vi "GVSDV DOCKING.vi"(8 "sData":string, 9 "DataView Index":i32, 11 "sAction":string) -> (0 "nData_Out":i32, 1 "tWindow_Out":T3, 2 "pVIRef_Tmp":refnum<vi>, 3 "pSPRef_Out":refnum<vi>)   [LabVIEW 2013]
uses:
  <vilib>/Utility/miscctls.llb/LVBoundsTypeDef.ctl
  <vilib>/Utility/miscctls.llb/LVPositionTypeDef.ctl
  GVSNew View Global.vi
panel:
  in  "child_sp_count":i32
  in  "spliter_idx":i32
  out "Position tmp":T1
  out "Container Bounds tmp":T2
  in  "cur_panel_idx":i32
  in  "pSPRef":refnum<vi>
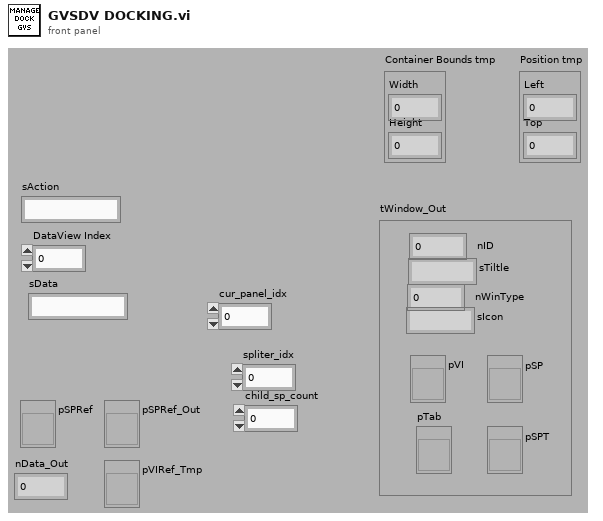
[diagram p1: front panel]
types:
  T1 = typedef "LVPositionTypeDef.ctl" = cluster{"Left":i32, "Top":i32}
  T2 = typedef "LVBoundsTypeDef.ctl" = cluster{"Width":u32, "Height":u32}
  T3 = cluster{"nID":i32, "sTiltle":string, "pVI":refnum<vi>, "pSP":refnum<vi>, "pTab":refnum<vi>, "pSPT":refnum<vi>, "nWinType":i32, "sIcon":string}
  T4 = typedef "Graph Main Info Cluster.ctl" = cluster{"Selected_BarIdx":i32, "Selected_PanelIdx":i32, "Graph Main VIRef":refnum<vi>, "ToolBarClick":bool, "Spliter Ref Array":refnum<vi>[], "Panel Ref Array":refnum<vi>[], "Spliter_matrix":i32[][], "Panel_matrix":i32[][], "child_spliterIdx_matrix":i32[][], "split_pos_matrix":i32[][], "Title State":bool, "sQueueName":string, "Frame nID":i32, "Graph VIRef Array":cluster{"Graph VIRef":refnum<vi>, "Panel Idx":i32, "Frame VIRef":refnum<vi>, "Icon Ring":i32, "Graph Type":string}[], "View Type":string}
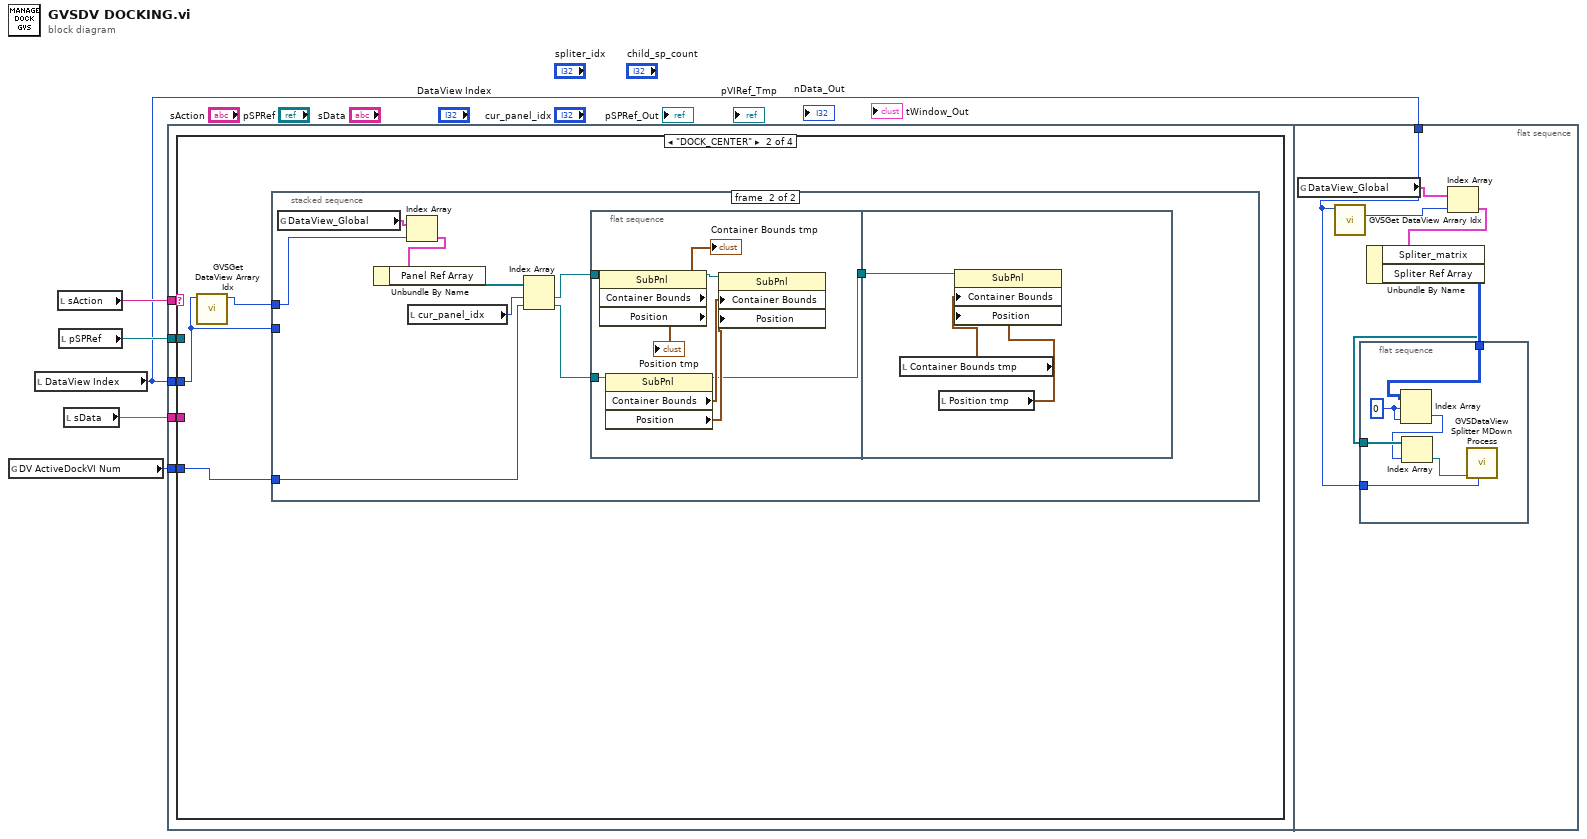
[diagram p0: block diagram]
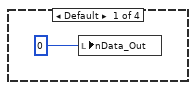
[diagram p2: hidden frame]
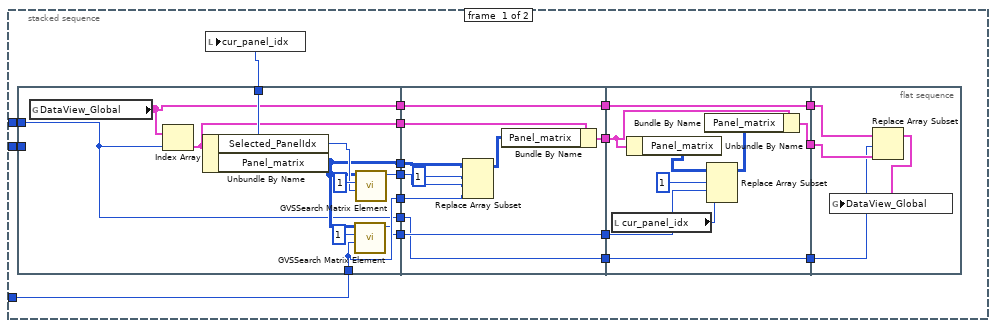
[diagram p3: hidden frame]
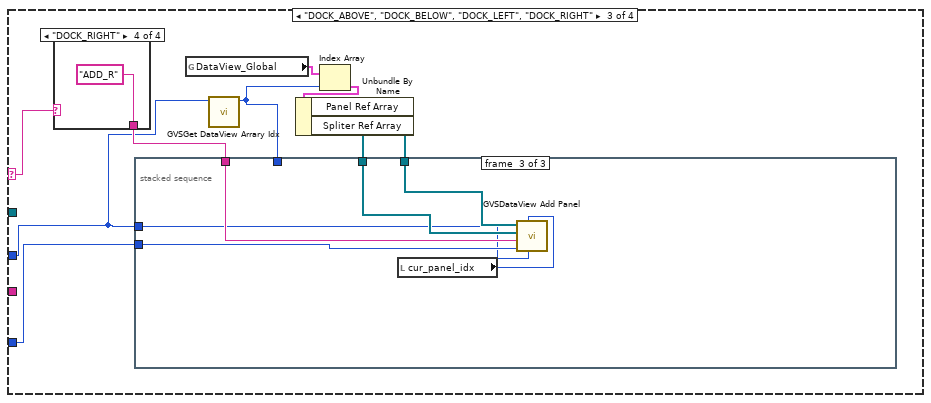
[diagram p4: hidden frame]
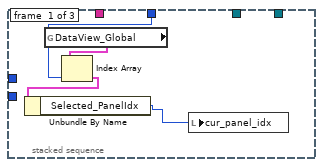
[diagram p5: hidden frame]
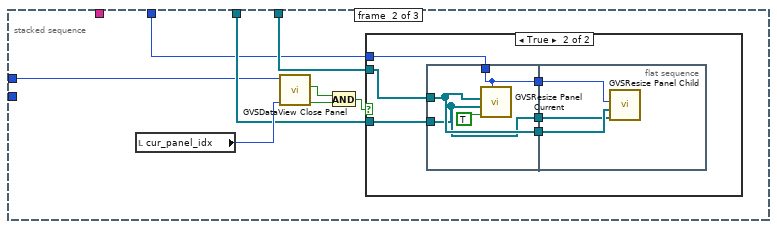
[diagram p6: hidden frame]
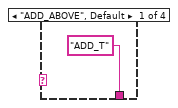
[diagram p8: hidden frame]
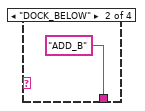
[diagram p9: hidden frame]
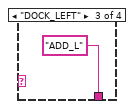
[diagram p10: hidden frame]
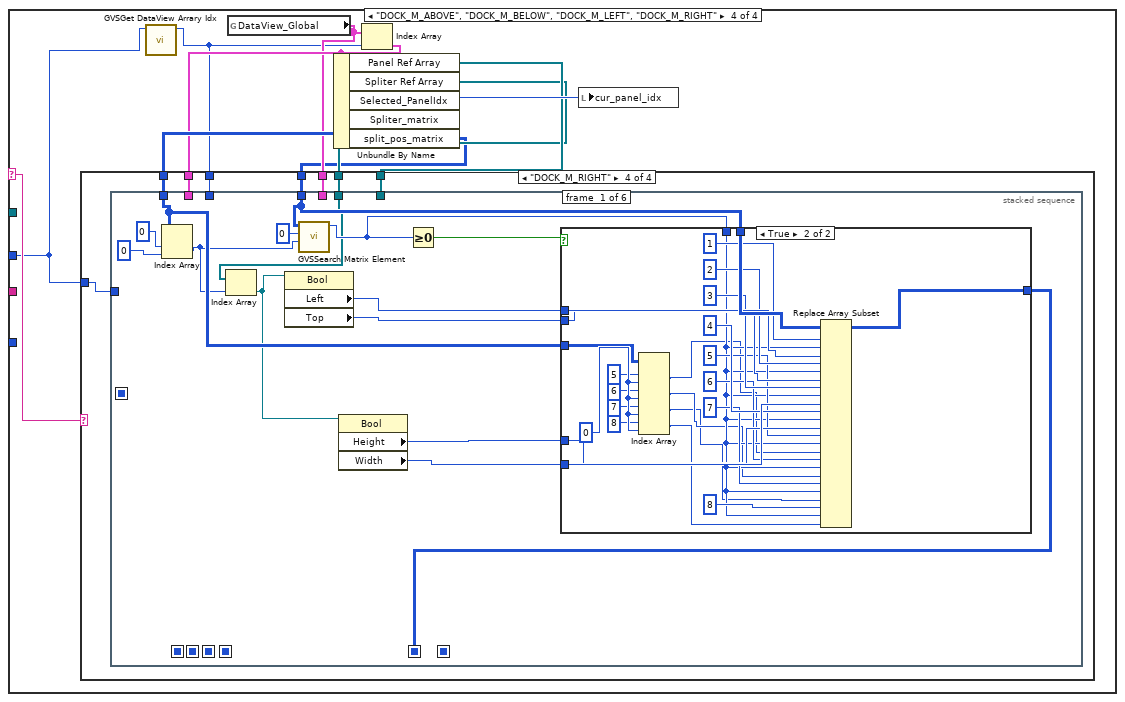
[diagram p11: hidden frame]
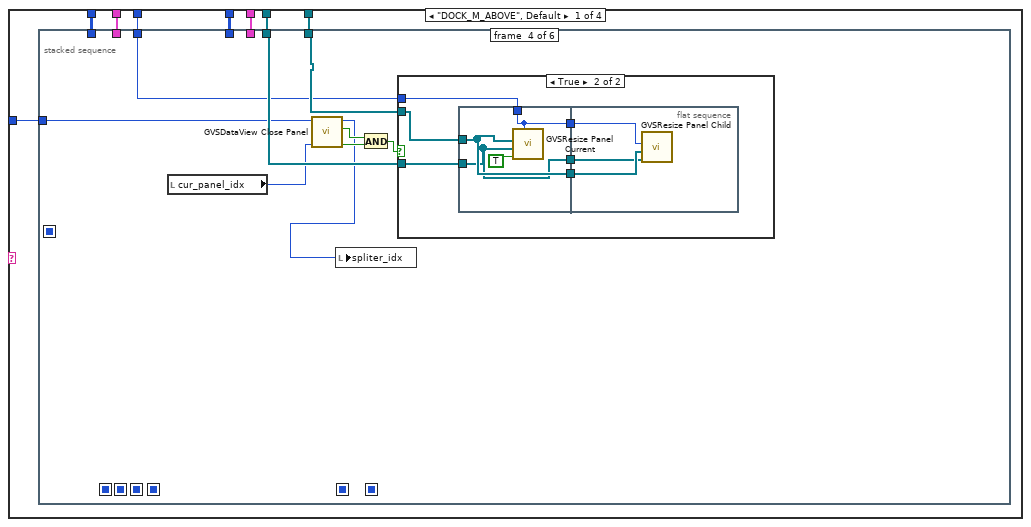
[diagram p12: hidden frame]
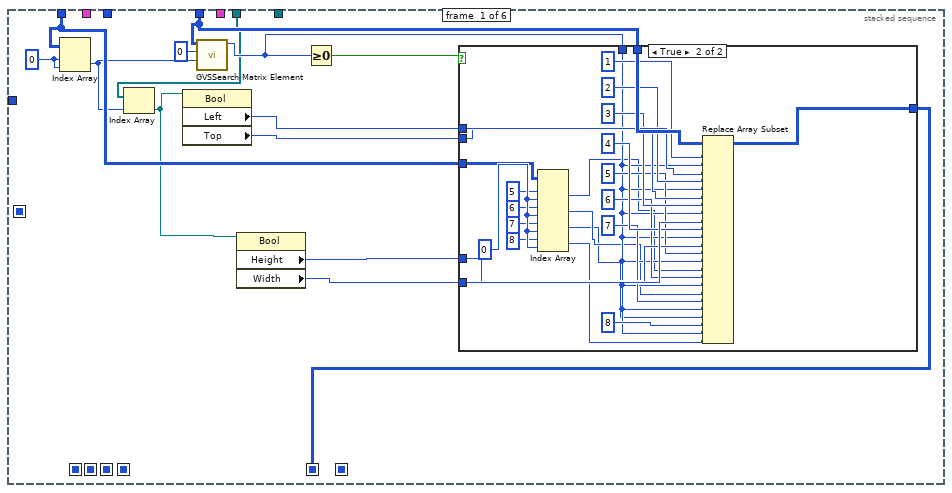
[diagram p13: hidden frame]
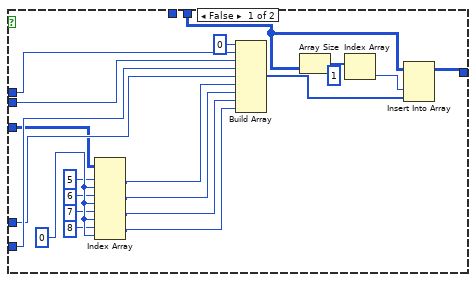
[diagram p14: hidden frame]
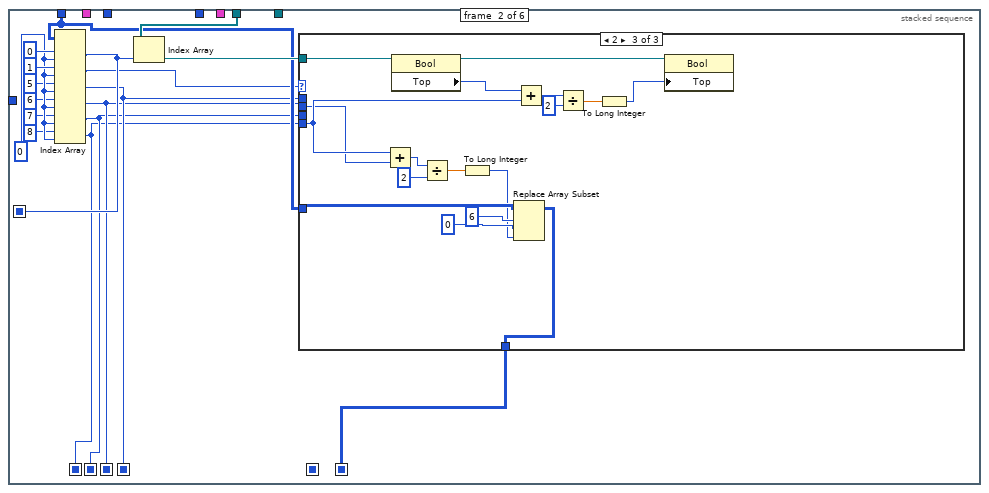
[diagram p15: hidden frame]
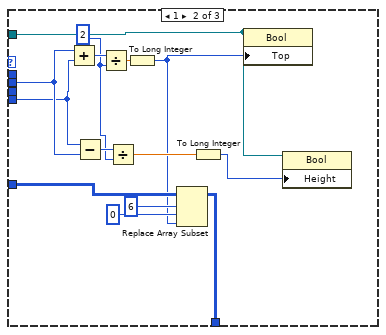
[diagram p17: hidden frame]
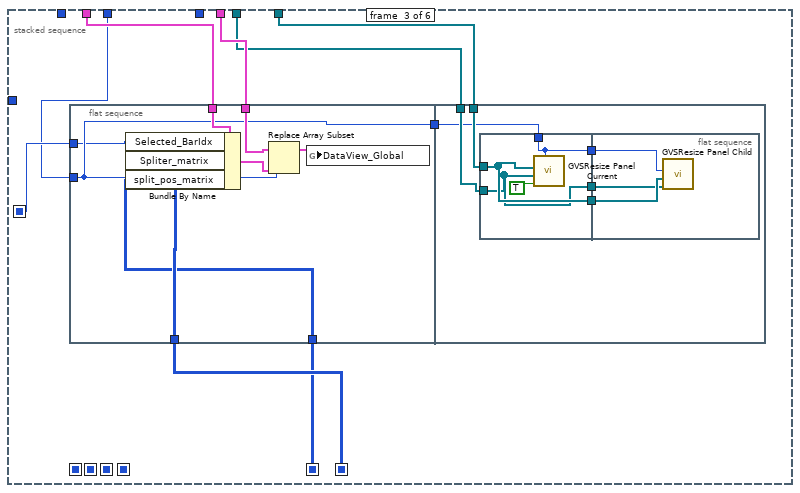
[diagram p18: hidden frame]
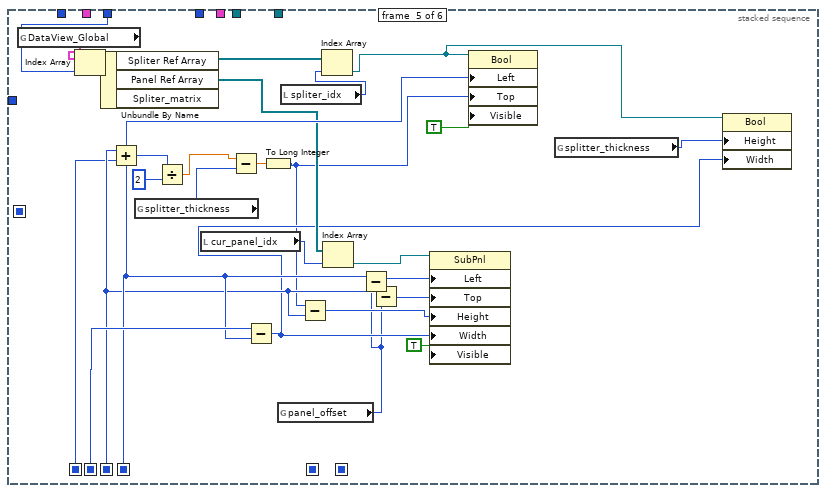
[diagram p20: hidden frame]
diagram:
  n1 = global read "GVSNew View Global.vi" "DV ActiveDockVI Num"() -> (w2:i32)
  n2 = local read "DataView Index"() -> (w1:i32)
  n3 = local read "sAction"() -> (w5:string)
  n4 = local read "pSPRef"() -> (w3:refnum<vi>)
  n5 = local read "sData"() -> (w4:string)
  n6 = flat-sequence {
    tunnel: w5 -> [w10]
    tunnel: w4 -> [w9]
    tunnel: w3 -> [w8]
    tunnel: w1 -> [w7]
    tunnel: w2 -> [w6]
    tunnel: w1 -> [w1261]
    frame #0 {
      n7 = case shown="\"DOCK_CENTER\"" w10 {
        selector: w10 -> [_ _ w94 w132]
        tunnel: w9 -> [_ _ _ _]
        tunnel: w8 -> [_ _ _ _]
        tunnel: w7 -> [_ w13 w86 w130]
        tunnel: w6 -> [_ w14 w93 _]
        frame Default {
          n8 = local write "nData_Out"(0 ("nData_Out")) -> ()
        }
        frame "DOCK_CENTER" {
          n9 = call "GVSGet DataView Arrary Idx.vi"("DataView Idx In"=w13) -> ("DataView Arrary Idx out"=w12:i32)  [unwired: 10 in]
          n10 = stacked-sequence {
            tunnel: w13 -> [w18 _]
            tunnel: w14 -> [w16 w72]
            tunnel: w12 -> [w15 w66]
            frame #0 {
              n11 = flat-sequence {
                tunnel: w18 -> [_]
                tunnel: [w41] -> w17
                tunnel: w16 -> [w37]
                tunnel: [w39] -> w32
                tunnel: [w38] -> w31
                tunnel: [w37] -> w30
                tunnel: [w36] -> w29
                tunnel: [w35] -> w28
                tunnel: [w34] -> w27
                tunnel: [w33] -> w26
                tunnel: w15 -> [w33]
                tunnel: w32 -> [w45]
                tunnel: w31 -> [w47]
                tunnel: w30 -> [w44]
                tunnel: w29 -> [w52]
                tunnel: [w51] -> w25
                tunnel: [w50] -> w24
                tunnel: w28 -> [w50]
                tunnel: [w49] -> w23
                tunnel: w27 -> [w49]
                tunnel: [w48] -> w22
                tunnel: w26 -> [w48]
                tunnel: w25 -> [w61]
                tunnel: w24 -> [w55]
                tunnel: [w60] -> w21
                tunnel: [w59] -> w20
                tunnel: w23 -> [w59]
                tunnel: [w58] -> w19
                tunnel: w22 -> [w58]
                tunnel: w21 -> [w64]
                tunnel: w20 -> [w65]
                tunnel: w19 -> [w63]
                frame #0 {
                  n12 = global read "GVSNew View Global.vi" "DataView_Global"() -> (w34:T4[])
                  n13 = Index Array(array=w34, index=w33) -> (element=w36:T4)
                  n14 = Unbundle By Name(w36) -> ("Selected_PanelIdx"=w41:i32, "Panel_matrix"=w38:i32[][])
                  n15 = call "GVSSearch Matrix Element.vi"("element"=w37, "index (row)"=1, "matrix in"=w38) -> ("index of element"=w35:i32)  [unwired: 8 in]
                  n16 = call "GVSSearch Matrix Element.vi"("element"=w41, "index (row)"=1, "matrix in"=w38) -> ("index of element"=w39:i32)  [unwired: 8 in]
                }
                frame #1 {
                  n17 = Replace Array Subset(array=w47, new element=w44, index (row)=1 ("disabled index (row)"), index (col)=w45) -> (w43:i32[][])
                  n18 = Bundle By Name(cluster=w52, "Panel_matrix"=w43) -> (w51:T4)
                }
                frame #2 {
                  n19 = local read "cur_panel_idx"() -> (w54:i32)
                  n20 = Unbundle By Name(w61) -> ("Panel_matrix"=w57:i32[][])
                  n21 = Replace Array Subset(array=w57, new element=w54, index (row)=1 ("disabled index (row)"), index (col)=w55) -> (w53:i32[][])
                  n22 = Bundle By Name(cluster=w61, "Panel_matrix"=w53) -> (w60:T4)
                }
                frame #3 {
                  n23 = Replace Array Subset(array=w65, new element=w64, index=w63) -> (w62:T4[])
                  n24 = global write "GVSNew View Global.vi" "DataView_Global"(w62) -> ()
                }
              }
              n25 = local write "cur_panel_idx"(w17) -> ()
            }
            frame #1 {
              n26 = global read "GVSNew View Global.vi" "DataView_Global"() -> (w69:T4[])
              n27 = Index Array(array=w69, index=w66) -> (element=w68:T4)
              n28 = Unbundle By Name(w68) -> ("Panel Ref Array"=w67:refnum<vi>[])
              n29 = local read "cur_panel_idx"() -> (w74:i32)
              n30 = Index Array(array=w67, index #1=w74, index #2=w72) -> (element #1=w73:refnum<vi>, element #2=w71:refnum<vi>)
              n31 = flat-sequence {
                tunnel: w73 -> [w82]
                tunnel: w71 -> [w78]
                tunnel: [w75] -> w70
                tunnel: w70 -> [w85]
                frame #0 {
                  n32 = property class="SubPnl"(reference=w82) -> (reference out=w79:refnum<vi>, "Container Bounds"=→"Container Bounds tmp":T2, "Position"=→"Position tmp":T1)  [unwired: 1 in, 1 out]
                  n33 = property class="SubPnl"(reference=w78) -> (reference out=w75:refnum<vi>, "Container Bounds"=w77:T2, "Position"=w76:T1)  [unwired: 1 in, 1 out]
                  n34 = property class="SubPnl"(reference=w79, "Container Bounds"=w77, "Position"=w76) -> ()  [unwired: 1 in, 2 out]
                }
                frame #1 {
                  n35 = local read "Container Bounds tmp"() -> (w84:T2)
                  n36 = local read "Position tmp"() -> (w83:T1)
                  n37 = property class="SubPnl"(reference=w85, "Container Bounds"=w84, "Position"=w83) -> ()  [unwired: 1 in, 2 out]
                }
              }
            }
          }
        }
        frame "DOCK_ABOVE", "DOCK_BELOW", "DOCK_LEFT", "DOCK_RIGHT" {
          n38 = case shown="\"DOCK_RIGHT\"" w94 {
            tunnel: ["ADD_T" "ADD_B" "ADD_L" "ADD_R"] -> w92
            frame "ADD_ABOVE", Default {
            }
            frame "DOCK_BELOW" {
            }
            frame "DOCK_LEFT" {
            }
            frame "DOCK_RIGHT" {
            }
          }
          n39 = global read "GVSNew View Global.vi" "DataView_Global"() -> (w91:T4[])
          n40 = call "GVSGet DataView Arrary Idx.vi"("DataView Idx In"=w86) -> ("DataView Arrary Idx out"=w87:i32)  [unwired: 10 in]
          n41 = Index Array(array=w91, index=w87) -> (element=w90:T4)
          n42 = Unbundle By Name(w90) -> ("Panel Ref Array"=w89:refnum<vi>[], "Spliter Ref Array"=w88:refnum<vi>[])
          n43 = stacked-sequence {
            tunnel: w93 -> [_ _ w125]
            tunnel: w92 -> [_ _ w124]
            tunnel: w89 -> [_ w102 w122]
            tunnel: w88 -> [_ w101 w121]
            tunnel: w87 -> [w95 w100 _]
            tunnel: w86 -> [_ w99 w120]
            frame #0 {
              n44 = global read "GVSNew View Global.vi" "DataView_Global"() -> (w97:T4[])
              n45 = Index Array(array=w97, index=w95) -> (element=w98:T4)
              n46 = Unbundle By Name(w98) -> ("Selected_PanelIdx"=w96:i32)
              n47 = local write "cur_panel_idx"(w96) -> ()
            }
            frame #1 {
              n48 = local read "cur_panel_idx"() -> (w103:i32)
              n49 = call "GVSDataView Close Panel.vi"("Panel_Idx"=w103, "DataView Index"=w99) -> ("bResult"=w105:bool, "bHaveChild"=w106:bool)  [unwired: 7 in, 1 out]
              n50 = And(x=w106, y=w105) -> (x .and. y?=w104:bool)
              n51 = case shown="True" w104 {
                tunnel: w102 -> [_ w112]
                tunnel: w101 -> [_ w111]
                tunnel: w100 -> [_ w110]
                frame False {
                }
                frame True {
                  n52 = flat-sequence {
                    tunnel: w112 -> [w114]
                    tunnel: w111 -> [w113]
                    tunnel: w110 -> [w115]
                    tunnel: [w115] -> w109
                    tunnel: [w114] -> w108
                    tunnel: [w113] -> w107
                    tunnel: w109 -> [w119]
                    tunnel: w108 -> [w118]
                    tunnel: w107 -> [w117]
                    frame #0 {
                      n53 = call "GVSResize Panel Current.vi"("DataView Array Idx"=w115, "close_panel"=TRUE, "spliter array"=w113, "SubPanel array"=w114) -> ()  [unwired: 8 in]
                    }
                    frame #1 {
                      n54 = call "GVSResize Panel Child.vi"("spliter array"=w117, "SubPanel array"=w118, "DataView Array Idx"=w119) -> ()  [unwired: 9 in]
                    }
                  }
                }
              }
            }
            frame #2 {
              n55 = local read "cur_panel_idx"() -> (w123:i32)
              n56 = call "GVSDataView Add Panel.vi"("DataView Index"=w120, "panel_index"=w123, "Selected Panel Idx"=w125, "SAdd_Pos"=w124, "spliter array"=w121, "SubPanel array"=w122) -> ()  [unwired: 3 in, 3 out]
            }
          }
        }
        frame "DOCK_M_ABOVE", "DOCK_M_BELOW", "DOCK_M_LEFT", "DOCK_M_RIGHT" {
          n57 = call "GVSGet DataView Arrary Idx.vi"("DataView Idx In"=w130) -> ("DataView Arrary Idx out"=w131:i32)  [unwired: 10 in]
          n58 = global read "GVSNew View Global.vi" "DataView_Global"() -> (w134:T4[])
          n59 = Index Array(array=w134, index=w131) -> (element=w135:T4)
          n60 = Unbundle By Name(w135) -> ("Panel Ref Array"=w138:refnum<vi>[], "Spliter Ref Array"=w137:refnum<vi>[], "Selected_PanelIdx"=w139:i32, "Spliter_matrix"=w136:i32[][], "split_pos_matrix"=w133:i32[][])
          n61 = case shown="\"DOCK_M_RIGHT\"" w132 {
            tunnel: w138 -> [w147 w427 w707 w988]
            tunnel: w137 -> [w146 w426 w706 w987]
            tunnel: w136 -> [w145 w425 w705 w986]
            tunnel: w135 -> [w144 w424 w704 w985]
            tunnel: w134 -> [w143 w423 w703 w984]
            tunnel: w133 -> [w142 w422 w702 w983]
            tunnel: w131 -> [w141 w421 w701 w981]
            tunnel: w130 -> [w140 w420 w700 w982]
            frame "DOCK_M_ABOVE", Default {
              n62 = stacked-sequence {
                seq-local: [_ w221 _ _ _ _] -> [_ _ w259 _ _ _]
                seq-local: [w152 _ _ _ _ _] -> [_ _ w258 _ _ _]
                seq-local: [_ w207 _ _ _ _] -> [_ _ _ _ w331 w345]
                seq-local: [_ w208 _ _ _ _] -> [_ _ _ _ w334 w346]
                seq-local: [_ w209 _ _ _ _] -> [_ _ _ _ w332 w347]
                seq-local: [_ w210 _ _ _ _] -> [_ _ _ _ w333 w348]
                seq-local: [_ w212 _ _ _ _] -> [_ _ w257 _ _ _]
                tunnel: w147 -> [_ _ w262 w293 _ _]
                tunnel: w146 -> [w157 w223 w261 w294 _ _]
                tunnel: w145 -> [w151 w213 _ _ _ _]
                tunnel: w144 -> [_ _ w264 _ _ _]
                tunnel: w143 -> [_ _ w263 _ _ _]
                tunnel: w142 -> [w158 _ _ _ _ _]
                tunnel: w141 -> [_ _ w256 w287 w316 w335]
                tunnel: w140 -> [_ _ _ w286 _ _]
                frame #0 {
                  w150 = 0 ("index (row)")
                  n63 = Index Array(array=w151, index (row)=w150, index (col)=w150) -> (element=w149:i32)
                  n64 = Index Array(array=w157, index=w149) -> (element=w148:refnum<vi>)
                  n65 = property class="Bool"(reference=w148) -> ("Left"=w156:i32, "Top"=w155:i32)  [unwired: 1 in, 2 out]
                  n66 = call "GVSSearch Matrix Element.vi"("element"=w149, "index (row)"=0, "matrix in"=w158) -> ("index of element"=w159:i32)  [unwired: 8 in]
                  n67 = property class="Bool"(reference=w148) -> ("Height"=w153:u32, "Width"=w154:u32)  [unwired: 1 in, 2 out]
                  n68 = Greater Or Equal To 0?(x=w159) -> (x >= 0?=w160:bool)
                  n69 = case shown="True" w160 {
                    tunnel: w159 -> [_ w193]
                    tunnel: w158 -> [w164 w206]
                    tunnel: w151 -> [w171 w186]
                    tunnel: w156 -> [w181 w204]
                    tunnel: w155 -> [w180 w202]
                    tunnel: w154 -> [w179 w200]
                    tunnel: w153 -> [w178 w198]
                    tunnel: [w162 w192] -> w152
                    frame False {
                      (unwired) 1 ("index")
                      w176 = 0 ("index (col)")
                      n70 = Index Array(array=w171, index (row) #1=5 ("index (row)"), index (col) #1=w176, index (row) #2=6 ("index (row)"), index (col) #2=w176, index (row) #3=7 ("index (row)"), index (col) #3=w176, index (row) #4=8 ("index (row)"), index (col) #4=w176) -> (element #1=w170:i32, element #2=w169:i32, element #3=w168:i32, element #4=w167:i32)
                      n71 = Build Array(0 ("element"), w181, w180, w179, w178, w170, w169, w168, w167) -> (w165:u32[])
                      n72 = Array Size(array=w164) -> (size(s)=w166:i32[])
                      n73 = Index Array(array=w166) -> (element=w163:i32)  [unwired: 1 in]
                      n74 = Insert Into Array(array=w164, index (col)=w163, new element=w165) -> (w162:i32[][])  [unwired: 1 in]
                    }
                    frame True {
                      w191 = 0 ("index (col)")
                      n75 = Index Array(array=w186, index (row) #1=5 ("index (row)"), index (col) #1=w191, index (row) #2=6 ("index (row)"), index (col) #2=w191, index (row) #3=7 ("index (row)"), index (col) #3=w191, index (row) #4=8 ("index (row)"), index (col) #4=w191) -> (element #1=w185:i32, element #2=w184:i32, element #3=w183:i32, element #4=w182:i32)
                      n76 = Replace Array Subset(array=w206, new element #1=w204, index (row) #1=1 ("disabled index (row)"), index (col) #1=w193, new element #2=w202, index (row) #2=2 ("disabled index (row)"), index (col) #2=w193, new element #3=w200, index (row) #3=3 ("disabled index (row)"), index (col) #3=w193, new element #4=w198, index (row) #4=4 ("disabled index (row)"), index (col) #4=w193, new element #5=w185, index (row) #5=5 ("disabled index (row)"), index (col) #5=w193, new element #6=w184, index (row) #6=6 ("disabled index (row)"), index (col) #6=w193, new element #7=w183, index (row) #7=7 ("disabled index (row)"), index (col) #7=w193, new element #8=w182, index (row) #8=8 ("disabled index (row)"), index (col) #8=w193) -> (w192:i32[][])
                    }
                  }
                }
                frame #1 {
                  w218 = 0 ("index (col)")
                  n77 = Index Array(array=w213, index (row) #1=0 ("index (row)"), index (col) #1=w218, index (row) #2=1 ("index (row)"), index (col) #2=w218, index (row) #3=5 ("index (row)"), index (col) #3=w218, index (row) #4=6 ("index (row)"), index (col) #4=w218, index (row) #5=7 ("index (row)"), index (col) #5=w218, index (row) #6=8 ("index (row)"), index (col) #6=w218) -> (element #1=w212:i32, element #2=w211:i32, element #3=w210:i32, element #4=w209:i32, element #5=w208:i32, element #6=w207:i32)
                  n78 = Index Array(array=w223, index=w212) -> (element=w222:refnum<vi>)
                  n79 = case shown="2" w211 {
                    tunnel: w222 -> [_ w225 w255]
                    tunnel: w210 -> [_ _ _]
                    tunnel: w209 -> [_ w235 w247]
                    tunnel: w208 -> [_ _ _]
                    tunnel: w207 -> [_ w234 w248]
                    tunnel: w213 -> [w224 w230 w246]
                    tunnel: [w224 w226 w243] -> w221
                    frame 0, Default {
                    }
                    frame 1 {
                      w236 = 2 ("y")
                      n80 = Add(x=w235, y=w234) -> (x+y=w238:i32)
                      n81 = Subtract(x=w234, y=w235) -> (x-y=w237:i32)
                      n82 = Divide(x=w238, y=w236) -> (x/y=w233:dbl)
                      n83 = Divide(x=w237, y=w236) -> (x/y=w232:dbl)
                      n84 = To Long Integer(number=w233) -> (32bit integer=w227:i32)
                      n85 = Replace Array Subset(array=w230, new element=w227, index (row)=6 ("disabled index (row)"), index (col)=0) -> (w226:i32[][])
                      n86 = To Long Integer(number=w232) -> (32bit integer=w231:i32)
                      n87 = property class="Bool"(reference=w225, "Top"=w227) -> ()  [unwired: 1 in, 2 out]
                      n88 = property class="Bool"(reference=w225, "Height"=w231) -> ()  [unwired: 1 in, 2 out]
                    }
                    frame 2 {
                      n89 = Add(x=w248, y=w247) -> (x+y=w250:i32)
                      n90 = property class="Bool"(reference=w255) -> (reference out=w254:refnum<vi>, "Top"=w251:i32)  [unwired: 1 in, 1 out]
                      n91 = Divide(x=w250, y=2) -> (x/y=w242:dbl)
                      n92 = To Long Integer(number=w242) -> (32bit integer=w241:i32)
                      n93 = Replace Array Subset(array=w246, new element=w241, index (row)=6 ("disabled index (row)"), index (col)=0) -> (w243:i32[][])
                      n94 = Add(x=w251, y=w248) -> (x+y=w253:i32)
                      n95 = Divide(x=w253, y=2) -> (x/y=w240:dbl)
                      n96 = To Long Integer(number=w240) -> (32bit integer=w239:i32)
                      n97 = property class="Bool"(reference=w254, "Top"=w239) -> ()  [unwired: 1 in, 2 out]
                    }
                  }
                }
                frame #2 {
                  n98 = flat-sequence {
                    tunnel: w264 -> [w272]
                    tunnel: w263 -> [w270]
                    tunnel: w256 -> [w268]
                    tunnel: [w268] -> w260
                    tunnel: w259 -> [w267]
                    tunnel: w258 -> [w266]
                    tunnel: w257 -> [w265]
                    tunnel: w262 -> [w275]
                    tunnel: w261 -> [w274]
                    tunnel: w260 -> [w273]
                    frame #0 {
                      n99 = Bundle By Name(cluster=w272, "Selected_BarIdx"=w265, "Spliter_matrix"=w267, "split_pos_matrix"=w266) -> (w271:T4)
                      n100 = Replace Array Subset(array=w270, new element=w271, index=w268) -> (w269:T4[])
                      n101 = global write "GVSNew View Global.vi" "DataView_Global"(w269) -> ()
                    }
                    frame #1 {
                      n102 = flat-sequence {
                        tunnel: w275 -> [w280]
                        tunnel: w274 -> [w279]
                        tunnel: w273 -> [w281]
                        tunnel: [w281] -> w278
                        tunnel: [w280] -> w277
                        tunnel: [w279] -> w276
                        tunnel: w278 -> [w285]
                        tunnel: w277 -> [w284]
                        tunnel: w276 -> [w283]
                        frame #0 {
                          n103 = call "GVSResize Panel Current.vi"("DataView Array Idx"=w281, "close_panel"=TRUE, "spliter array"=w279, "SubPanel array"=w280) -> ()  [unwired: 8 in]
                        }
                        frame #1 {
                          n104 = call "GVSResize Panel Child.vi"("spliter array"=w283, "SubPanel array"=w284, "DataView Array Idx"=w285) -> ()  [unwired: 9 in]
                        }
                      }
                    }
                  }
                }
                frame #3 {
                  n105 = local read "cur_panel_idx"() -> (w289:i32)
                  n106 = call "GVSDataView Close Panel.vi"("Panel_Idx"=w289, "DataView Index"=w286) -> ("bResult"=w291:bool, "bHaveChild"=w292:bool, "closed_spliter_idx"=w288:i32)  [unwired: 7 in]
                  n107 = local write "spliter_idx"(w288) -> ()
                  n108 = And(x=w292, y=w291) -> (x .and. y?=w290:bool)
                  n109 = case shown="True" w290 {
                    tunnel: w293 -> [_ w300]
                    tunnel: w294 -> [_ w299]
                    tunnel: w287 -> [_ w298]
                    frame False {
                    }
                    frame True {
                      n110 = flat-sequence {
                        tunnel: w300 -> [w302]
                        tunnel: w299 -> [w301]
                        tunnel: w298 -> [w303]
                        tunnel: [w303] -> w297
                        tunnel: [w302] -> w296
                        tunnel: [w301] -> w295
                        tunnel: w297 -> [w307]
                        tunnel: w296 -> [w306]
                        tunnel: w295 -> [w305]
                        frame #0 {
                          n111 = call "GVSResize Panel Current.vi"("DataView Array Idx"=w303, "close_panel"=TRUE, "spliter array"=w301, "SubPanel array"=w302) -> ()  [unwired: 8 in]
                        }
                        frame #1 {
                          n112 = call "GVSResize Panel Child.vi"("spliter array"=w305, "SubPanel array"=w306, "DataView Array Idx"=w307) -> ()  [unwired: 9 in]
                        }
                      }
                    }
                  }
                }
                frame #4 {
                  n113 = global read "GVSNew View Global.vi" "DataView_Global"() -> (w328:T4[])
                  n114 = Index Array(array=w328, index=w316) -> (element=w327:T4)
                  n115 = Unbundle By Name(w327) -> ("Spliter Ref Array"=w326:refnum<vi>[], "Panel Ref Array"=w325:refnum<vi>[])  [unwired: 1 out]
                  n116 = Add(x=w332, y=w331) -> (x+y=w320:i32)
                  n117 = global read "GVSNew View Global.vi" "splitter_thickness"() -> (w308:u32)
                  n118 = Divide(x=w320, y=2) -> (x/y=w318:dbl)
                  n119 = local read "cur_panel_idx"() -> (w324:i32)
                  n120 = Subtract(x=w318, y=w308) -> (x-y=w315:dbl)
                  n121 = Subtract(x=w334, y=w333) -> (x-y=w317:i32)
                  n122 = To Long Integer(number=w315) -> (32bit integer=w314:i32)
                  n123 = global read "GVSNew View Global.vi" "panel_offset"() -> (w310:i32)
                  n124 = local read "spliter_idx"() -> (w330:i32)
                  n125 = Subtract(x=w314, y=w332) -> (x-y=w322:i32)
                  n126 = Index Array(array=w326, index=w330) -> (element=w313:refnum<vi>)
                  n127 = Index Array(array=w325, index=w324) -> (element=w323:refnum<vi>)
                  n128 = Subtract(x=w333, y=w310) -> (x-y=w312:i32)
                  n129 = Subtract(x=w332, y=w310) -> (x-y=w311:i32)
                  n130 = property class="SubPnl"(reference=w323, "Left"=w312, "Top"=w311, "Height"=w322, "Width"=w317, "Visible"=TRUE) -> ()  [unwired: 1 in, 2 out]
                  n131 = property class="Bool"(reference=w313, "Left"=w333, "Top"=w314, "Visible"=TRUE) -> ()  [unwired: 1 in, 2 out]
                  n132 = global read "GVSNew View Global.vi" "splitter_thickness"() -> (w309:u32)
                  n133 = property class="Bool"(reference=w313, "Height"=w309, "Width"=w317) -> ()  [unwired: 1 in, 2 out]
                }
                frame #5 {
                  n134 = global read "GVSNew View Global.vi" "DataView_Global"() -> (w337:T4[])
                  n135 = Index Array(array=w337, index=w335) -> (element=w338:T4)
                  n136 = Unbundle By Name(w338) -> ("Spliter_matrix"=w344:i32[][], "Panel_matrix"=w339:i32[][], "child_spliterIdx_matrix"=w336:i32[][])  [unwired: 1 out]
                  n137 = Index Array(array=w344, index (row)=0) -> (element=w342:i32[])  [unwired: 1 in]
                  n138 = Array Size(array=w342) -> (size(s)=w341:i32)
                  n139 = Greater Than 0?(x=w341) -> (x > 0?=w340:bool)
                  n140 = case shown="True" w340 {
                    tunnel: w336 -> [w390 _]
                    tunnel: w348 -> [w384 w416]
                    tunnel: w347 -> [w383 w415]
                    tunnel: w346 -> [w382 w414]
                    tunnel: w345 -> [w381 w413]
                    tunnel: w344 -> [w354 w400]
                    tunnel: w339 -> [w363 w397]
                    tunnel: w336 -> [w365 _]
                    tunnel: w338 -> [w373 w408]
                    tunnel: w337 -> [w372 w407]
                    tunnel: w335 -> [w369 w404]
                    frame True {
                      w385 = -1 ("element")
                      w357 = 0 ("index (col)")
                      w351 = 0 ("index (col)")
                      n141 = Index Array(array=w354, index (row) #1=0 ("index (row)"), index (col) #1=w351, index (row) #2=3 ("index (row)"), index (col) #2=w351) -> (element #1=w349:i32, element #2=w350:i32)
                      n142 = local write "child_sp_count"(w350) -> ()
                      n143 = Index Array(array=w390, index (col)=w349) -> (element=w376:i32[])  [unwired: 1 in]
                      n144 = local read "child_sp_count"() -> (w387:i32)
                      n145 = Insert Into Array(array=w376, index=0, new element=w349) -> (w374:i32[])
                      n146 = Increment(x=w387) -> (x+1=w386:i32)
                      n147 = local read "spliter_idx"() -> (w359:i32)
                      n148 = local read "spliter_idx"() -> (w379:i32)
                      n149 = local read "cur_panel_idx"() -> (w378:i32)
                      n150 = Replace Array Subset(array=w354, new element #1=w359, index (row) #1=2 ("disabled index (row)"), index (col) #1=w357, new element #2=4 ("new element/submatrix"), index (row) #2=4 ("disabled index (row)"), index (col) #2=w357) -> (w355:i32[][])
                      n151 = Build Array(w379, 2 ("element"), w385, w386, w385, w384, w383, w382, w381) -> (w380:i32[])
                      n152 = Insert Into Array(array=w355, index (col)=0 ("disabled index (col)"), new element=w380) -> (w361:i32[][])  [unwired: 1 in]
                      n153 = Build Array(w379, w378, 3 ("element")) -> (w368:i32[])
                      n154 = local read "spliter_idx"() -> (w366:i32)
                      n155 = Insert Into Array(array=w363, index (col)=0 ("disabled index (col)"), new element=w368) -> (w362:i32[][])  [unwired: 1 in]
                      n156 = Replace Array Subset(array=w365, new element=w374, index (col)=w366) -> (w364:i32[][])  [unwired: 1 in]
                      n157 = Bundle By Name(cluster=w373, "Spliter_matrix"=w361, "Panel_matrix"=w362, "child_spliterIdx_matrix"=w364) -> (w370:T4)
                      n158 = Replace Array Subset(array=w372, new element=w370, index=w369) -> (w371:T4[])
                      n159 = global write "GVSNew View Global.vi" "DataView_Global"(w371) -> ()
                    }
                    frame False {
                      w393 = 0 ("index (col)")
                      w417 = -1 ("element")
                      n160 = local read "spliter_idx"() -> (w395:i32)
                      n161 = Replace Array Subset(array=w397, new element #1=w395, index (row) #1=0 ("disabled index (row)"), index (col) #1=w393, new element #2=4 ("new element/submatrix"), index (row) #2=2 ("disabled index (row)"), index (col) #2=w393) -> (w391:i32[][])
                      n162 = local read "spliter_idx"() -> (w411:i32)
                      n163 = local read "cur_panel_idx"() -> (w410:i32)
                      n164 = Build Array(w411, 2 ("element"), w417, 0 ("element"), w417, w416, w415, w414, w413) -> (w412:i32[])
                      n165 = Insert Into Array(array=w400, index (col)=0 ("disabled index (col)"), new element=w412) -> (w399:i32[][])  [unwired: 1 in]
                      n166 = Build Array(w411, w410, 3 ("element")) -> (w403:i32[])
                      n167 = Insert Into Array(array=w391, index (col)=0 ("disabled index (col)"), new element=w403) -> (w398:i32[][])  [unwired: 1 in]
                      n168 = Bundle By Name(cluster=w408, "Spliter_matrix"=w399, "Panel_matrix"=w398) -> (w405:T4)
                      n169 = Replace Array Subset(array=w407, new element=w405, index=w404) -> (w406:T4[])
                      n170 = global write "GVSNew View Global.vi" "DataView_Global"(w406) -> ()
                    }
                  }
                }
              }
            }
            frame "DOCK_M_BELOW" {
              n171 = stacked-sequence {
                seq-local: [_ w502 _ _ _ _] -> [_ _ w539 _ _ _]
                seq-local: [w433 _ _ _ _ _] -> [_ _ w538 _ _ _]
                seq-local: [_ w488 _ _ _ _] -> [_ _ _ _ w598 w625]
                seq-local: [_ w489 _ _ _ _] -> [_ _ _ _ w614 w626]
                seq-local: [_ w490 _ _ _ _] -> [_ _ _ _ w612 w627]
                seq-local: [_ w491 _ _ _ _] -> [_ _ _ _ w613 w628]
                seq-local: [_ w493 _ _ _ _] -> [_ _ w537 _ _ _]
                tunnel: w427 -> [_ _ w542 w573 _ _]
                tunnel: w426 -> [w438 w504 w541 w574 _ _]
                tunnel: w425 -> [w432 w494 _ _ _ _]
                tunnel: w424 -> [_ _ w544 _ _ _]
                tunnel: w423 -> [_ _ w543 _ _ _]
                tunnel: w422 -> [w439 _ _ _ _ _]
                tunnel: w421 -> [_ _ w536 w567 w596 w615]
                tunnel: w420 -> [_ _ _ w566 _ _]
                frame #0 {
                  n172 = Index Array(array=w432, index (row)=0, index (col)=0) -> (element=w429:i32)
                  n173 = Index Array(array=w438, index=w429) -> (element=w428:refnum<vi>)
                  n174 = property class="Bool"(reference=w428) -> ("Left"=w437:i32, "Top"=w436:i32)  [unwired: 1 in, 2 out]
                  n175 = call "GVSSearch Matrix Element.vi"("element"=w429, "index (row)"=0, "matrix in"=w439) -> ("index of element"=w440:i32)  [unwired: 8 in]
                  n176 = property class="Bool"(reference=w428) -> ("Height"=w434:u32, "Width"=w435:u32)  [unwired: 1 in, 2 out]
                  n177 = Greater Or Equal To 0?(x=w440) -> (x >= 0?=w441:bool)
                  n178 = case shown="True" w441 {
                    tunnel: w440 -> [_ w474]
                    tunnel: w439 -> [w445 w487]
                    tunnel: w432 -> [w450 w468]
                    tunnel: w437 -> [w462 w485]
                    tunnel: w436 -> [w461 w483]
                    tunnel: w435 -> [w460 w481]
                    tunnel: w434 -> [w459 w479]
                    tunnel: [w443 w463] -> w433
                    frame False {
                      (unwired) 1 ("index")
                      w457 = 0 ("index (col)")
                      n179 = Index Array(array=w450, index (row) #1=5 ("index (row)"), index (col) #1=w457, index (row) #2=6 ("index (row)"), index (col) #2=w457, index (row) #3=7 ("index (row)"), index (col) #3=w457, index (row) #4=8 ("index (row)"), index (col) #4=w457) -> (element #1=w452:i32, element #2=w451:i32, element #3=w449:i32, element #4=w448:i32)
                      n180 = Build Array(0 ("element"), w462, w461, w460, w459, w452, w451, w449, w448) -> (w444:u32[])
                      n181 = Array Size(array=w445) -> (size(s)=w446:i32[])
                      n182 = Index Array(array=w446) -> (element=w447:i32)  [unwired: 1 in]
                      n183 = Insert Into Array(array=w445, index (col)=w447, new element=w444) -> (w443:i32[][])  [unwired: 1 in]
                    }
                    frame True {
                      w473 = 0 ("index (col)")
                      n184 = Index Array(array=w468, index (row) #1=5 ("index (row)"), index (col) #1=w473, index (row) #2=6 ("index (row)"), index (col) #2=w473, index (row) #3=7 ("index (row)"), index (col) #3=w473, index (row) #4=8 ("index (row)"), index (col) #4=w473) -> (element #1=w467:i32, element #2=w466:i32, element #3=w465:i32, element #4=w464:i32)
                      n185 = Replace Array Subset(array=w487, new element #1=w485, index (row) #1=1 ("disabled index (row)"), index (col) #1=w474, new element #2=w483, index (row) #2=2 ("disabled index (row)"), index (col) #2=w474, new element #3=w481, index (row) #3=3 ("disabled index (row)"), index (col) #3=w474, new element #4=w479, index (row) #4=4 ("disabled index (row)"), index (col) #4=w474, new element #5=w467, index (row) #5=5 ("disabled index (row)"), index (col) #5=w474, new element #6=w466, index (row) #6=6 ("disabled index (row)"), index (col) #6=w474, new element #7=w465, index (row) #7=7 ("disabled index (row)"), index (col) #7=w474, new element #8=w464, index (row) #8=8 ("disabled index (row)"), index (col) #8=w474) -> (w463:i32[][])
                    }
                  }
                }
                frame #1 {
                  w499 = 0 ("index (col)")
                  n186 = Index Array(array=w494, index (row) #1=0 ("index (row)"), index (col) #1=w499, index (row) #2=1 ("index (row)"), index (col) #2=w499, index (row) #3=5 ("index (row)"), index (col) #3=w499, index (row) #4=6 ("index (row)"), index (col) #4=w499, index (row) #5=7 ("index (row)"), index (col) #5=w499, index (row) #6=8 ("index (row)"), index (col) #6=w499) -> (element #1=w493:i32, element #2=w492:i32, element #3=w491:i32, element #4=w490:i32, element #5=w489:i32, element #6=w488:i32)
                  n187 = Index Array(array=w504, index=w493) -> (element=w503:refnum<vi>)
                  n188 = case shown="1" w492 {
                    tunnel: w503 -> [_ w506 w535]
                    tunnel: w491 -> [_ _ _]
                    tunnel: w490 -> [_ w514 w527]
                    tunnel: w489 -> [_ _ _]
                    tunnel: w488 -> [_ w515 w528]
                    tunnel: w494 -> [w505 w513 w524]
                    tunnel: [w505 w509 w519] -> w502
                    frame 0, Default {
                    }
                    frame 1 {
                      w516 = 2 ("y")
                      n189 = Add(x=w514, y=w515) -> (x+y=w518:i32)
                      n190 = Subtract(x=w515, y=w514) -> (x-y=w517:i32)
                      n191 = Divide(x=w518, y=w516) -> ()  [unwired: 1 out]
                      n192 = Divide(x=w517, y=w516) -> (x/y=w508:dbl)
                      n193 = To Long Integer(number=w508) -> (32bit integer=w507:i32)
                      n194 = Add(x=w514, y=w507) -> (x+y=w510:i32)
                      n195 = Replace Array Subset(array=w513, new element=w510, index (row)=8 ("disabled index (row)"), index (col)=0) -> (w509:i32[][])
                      n196 = property class="Bool" props=["Top"](reference=w506) -> ()  [unwired: 1 in, 3 out]
                      n197 = property class="Bool"(reference=w506, "Height"=w507) -> ()  [unwired: 1 in, 2 out]
                    }
                    frame 2 {
                      n198 = Add(x=w528, y=w527) -> (x+y=w530:i32)
                      n199 = property class="Bool"(reference=w535) -> (reference out=w534:refnum<vi>, "Top"=w531:i32)  [unwired: 1 in, 1 out]
                      n200 = Divide(x=w530, y=2.0) -> (x/y=w521:dbl)
                      n201 = To Long Integer(number=w521) -> (32bit integer=w520:i32)
                      n202 = Replace Array Subset(array=w524, new element=w520, index (row)=8 ("disabled index (row)"), index (col)=0) -> (w519:i32[][])
                      n203 = Add(x=w531, y=w527) -> (x+y=w533:i32)
                      n204 = Divide(x=w533, y=2) -> (x/y=w526:dbl)
                      n205 = To Long Integer(number=w526) -> (32bit integer=w525:i32)
                      n206 = property class="Bool"(reference=w534, "Top"=w525) -> ()  [unwired: 1 in, 2 out]
                    }
                  }
                }
                frame #2 {
                  n207 = flat-sequence {
                    tunnel: w544 -> [w552]
                    tunnel: w543 -> [w550]
                    tunnel: w536 -> [w548]
                    tunnel: [w548] -> w540
                    tunnel: w539 -> [w547]
                    tunnel: w538 -> [w546]
                    tunnel: w537 -> [w545]
                    tunnel: w542 -> [w555]
                    tunnel: w541 -> [w554]
                    tunnel: w540 -> [w553]
                    frame #0 {
                      n208 = Bundle By Name(cluster=w552, "Selected_BarIdx"=w545, "Spliter_matrix"=w547, "split_pos_matrix"=w546) -> (w551:T4)
                      n209 = Replace Array Subset(array=w550, new element=w551, index=w548) -> (w549:T4[])
                      n210 = global write "GVSNew View Global.vi" "DataView_Global"(w549) -> ()
                    }
                    frame #1 {
                      n211 = flat-sequence {
                        tunnel: w555 -> [w560]
                        tunnel: w554 -> [w559]
                        tunnel: w553 -> [w561]
                        tunnel: [w561] -> w558
                        tunnel: [w560] -> w557
                        tunnel: [w559] -> w556
                        tunnel: w558 -> [w565]
                        tunnel: w557 -> [w564]
                        tunnel: w556 -> [w563]
                        frame #0 {
                          n212 = call "GVSResize Panel Current.vi"("DataView Array Idx"=w561, "close_panel"=TRUE, "spliter array"=w559, "SubPanel array"=w560) -> ()  [unwired: 8 in]
                        }
                        frame #1 {
                          n213 = call "GVSResize Panel Child.vi"("spliter array"=w563, "SubPanel array"=w564, "DataView Array Idx"=w565) -> ()  [unwired: 9 in]
                        }
                      }
                    }
                  }
                }
                frame #3 {
                  n214 = local read "cur_panel_idx"() -> (w569:i32)
                  n215 = call "GVSDataView Close Panel.vi"("Panel_Idx"=w569, "DataView Index"=w566) -> ("bResult"=w571:bool, "bHaveChild"=w572:bool, "closed_spliter_idx"=w568:i32)  [unwired: 7 in]
                  n216 = local write "spliter_idx"(w568) -> ()
                  n217 = And(x=w572, y=w571) -> (x .and. y?=w570:bool)
                  n218 = case shown="True" w570 {
                    tunnel: w573 -> [_ w580]
                    tunnel: w574 -> [_ w579]
                    tunnel: w567 -> [_ w578]
                    frame False {
                    }
                    frame True {
                      n219 = flat-sequence {
                        tunnel: w580 -> [w582]
                        tunnel: w579 -> [w581]
                        tunnel: w578 -> [w583]
                        tunnel: [w583] -> w577
                        tunnel: [w582] -> w576
                        tunnel: [w581] -> w575
                        tunnel: w577 -> [w587]
                        tunnel: w576 -> [w586]
                        tunnel: w575 -> [w585]
                        frame #0 {
                          n220 = call "GVSResize Panel Current.vi"("DataView Array Idx"=w583, "close_panel"=TRUE, "spliter array"=w581, "SubPanel array"=w582) -> ()  [unwired: 8 in]
                        }
                        frame #1 {
                          n221 = call "GVSResize Panel Child.vi"("spliter array"=w585, "SubPanel array"=w586, "DataView Array Idx"=w587) -> ()  [unwired: 9 in]
                        }
                      }
                    }
                  }
                }
                frame #4 {
                  n222 = global read "GVSNew View Global.vi" "DataView_Global"() -> (w609:T4[])
                  n223 = Index Array(array=w609, index=w596) -> (element=w608:T4)
                  n224 = Unbundle By Name(w608) -> ("Spliter Ref Array"=w607:refnum<vi>[], "Panel Ref Array"=w606:refnum<vi>[])  [unwired: 1 out]
                  n225 = Add(x=w612, y=w598) -> (x+y=w601:i32)
                  n226 = global read "GVSNew View Global.vi" "splitter_thickness"() -> (w588:u32)
                  n227 = Divide(x=w601, y=2) -> (x/y=w595:dbl)
                  n228 = To Long Integer(number=w595) -> (32bit integer=w594:i32)
                  n229 = local read "cur_panel_idx"() -> (w605:i32)
                  n230 = Add(x=w594, y=w588) -> (x+y=w597:u32)
                  n231 = Subtract(x=w614, y=w613) -> (x-y=w599:i32)
                  n232 = global read "GVSNew View Global.vi" "panel_offset"() -> (w590:i32)
                  n233 = local read "spliter_idx"() -> (w611:i32)
                  n234 = Subtract(x=w598, y=w597) -> (x-y=w603:u32)
                  n235 = Index Array(array=w607, index=w611) -> (element=w593:refnum<vi>)
                  n236 = Index Array(array=w606, index=w605) -> (element=w604:refnum<vi>)
                  n237 = Subtract(x=w613, y=w590) -> (x-y=w592:i32)
                  n238 = Subtract(x=w597, y=w590) -> (x-y=w591:u32)
                  n239 = property class="SubPnl"(reference=w604, "Left"=w592, "Top"=w591, "Height"=w603, "Width"=w599, "Visible"=TRUE) -> ()  [unwired: 1 in, 2 out]
                  n240 = property class="Bool"(reference=w593, "Left"=w613, "Top"=w594, "Visible"=TRUE) -> ()  [unwired: 1 in, 2 out]
                  n241 = global read "GVSNew View Global.vi" "splitter_thickness"() -> (w589:u32)
                  n242 = property class="Bool"(reference=w593, "Height"=w589, "Width"=w599) -> ()  [unwired: 1 in, 2 out]
                }
                frame #5 {
                  n243 = global read "GVSNew View Global.vi" "DataView_Global"() -> (w617:T4[])
                  n244 = Index Array(array=w617, index=w615) -> (element=w618:T4)
                  n245 = Unbundle By Name(w618) -> ("Spliter_matrix"=w624:i32[][], "Panel_matrix"=w619:i32[][], "child_spliterIdx_matrix"=w616:i32[][])  [unwired: 1 out]
                  n246 = Index Array(array=w624, index (row)=0) -> (element=w622:i32[])  [unwired: 1 in]
                  n247 = Array Size(array=w622) -> (size(s)=w621:i32)
                  n248 = Greater Than 0?(x=w621) -> (x > 0?=w620:bool)
                  n249 = case shown="False" w620 {
                    tunnel: w616 -> [w670 _]
                    tunnel: w628 -> [w664 w696]
                    tunnel: w627 -> [w663 w695]
                    tunnel: w626 -> [w662 w694]
                    tunnel: w625 -> [w661 w693]
                    tunnel: w624 -> [w634 w674]
                    tunnel: w619 -> [w643 w680]
                    tunnel: w616 -> [w645 _]
                    tunnel: w618 -> [w653 w688]
                    tunnel: w617 -> [w652 w687]
                    tunnel: w615 -> [w649 w684]
                    frame True {
                      w665 = -1 ("element")
                      w637 = 0 ("index (col)")
                      w631 = 0 ("index (col)")
                      n250 = Index Array(array=w634, index (row) #1=0 ("index (row)"), index (col) #1=w631, index (row) #2=3 ("index (row)"), index (col) #2=w631) -> (element #1=w629:i32, element #2=w630:i32)
                      n251 = local write "child_sp_count"(w630) -> ()
                      n252 = Index Array(array=w670, index (col)=w629) -> (element=w656:i32[])  [unwired: 1 in]
                      n253 = local read "child_sp_count"() -> (w667:i32)
                      n254 = Insert Into Array(array=w656, index=0, new element=w629) -> (w654:i32[])
                      n255 = Increment(x=w667) -> (x+1=w666:i32)
                      n256 = local read "spliter_idx"() -> (w639:i32)
                      n257 = local read "spliter_idx"() -> (w659:i32)
                      n258 = local read "cur_panel_idx"() -> (w658:i32)
                      n259 = Build Array(w659, 2 ("element"), w665, w666, w665, w664, w663, w662, w661) -> (w660:i32[])
                      n260 = Replace Array Subset(array=w634, new element #1=w639, index (row) #1=2 ("disabled index (row)"), index (col) #1=w637, new element #2=3 ("new element/submatrix"), index (row) #2=4 ("disabled index (row)"), index (col) #2=w637) -> (w635:i32[][])
                      n261 = Insert Into Array(array=w635, index (col)=0 ("disabled index (col)"), new element=w660) -> (w641:i32[][])  [unwired: 1 in]
                      n262 = Build Array(w659, w658, 4 ("element")) -> (w648:i32[])
                      n263 = local read "spliter_idx"() -> (w646:i32)
                      n264 = Insert Into Array(array=w643, index (col)=0 ("disabled index (col)"), new element=w648) -> (w642:i32[][])  [unwired: 1 in]
                      n265 = Replace Array Subset(array=w645, new element=w654, index (col)=w646) -> (w644:i32[][])  [unwired: 1 in]
                      n266 = Bundle By Name(cluster=w653, "Spliter_matrix"=w641, "Panel_matrix"=w642, "child_spliterIdx_matrix"=w644) -> (w650:T4)
                      n267 = Replace Array Subset(array=w652, new element=w650, index=w649) -> (w651:T4[])
                      n268 = global write "GVSNew View Global.vi" "DataView_Global"(w651) -> ()
                    }
                    frame False {
                      w676 = 0 ("index (col)")
                      w697 = -1 ("element")
                      n269 = local read "spliter_idx"() -> (w678:i32)
                      n270 = Replace Array Subset(array=w680, new element #1=w678, index (row) #1=0 ("disabled index (row)"), index (col) #1=w676, new element #2=3 ("new element/submatrix"), index (row) #2=2 ("disabled index (row)"), index (col) #2=w676) -> (w672:i32[][])
                      n271 = local read "spliter_idx"() -> (w691:i32)
                      n272 = local read "cur_panel_idx"() -> (w690:i32)
                      n273 = Build Array(w691, 2 ("element"), w697, 0 ("element"), w697, w696, w695, w694, w693) -> (w692:i32[])
                      n274 = Insert Into Array(array=w674, index (col)=0 ("disabled index (col)"), new element=w692) -> (w673:i32[][])  [unwired: 1 in]
                      n275 = Build Array(w691, w690, 4 ("element")) -> (w683:i32[])
                      n276 = Insert Into Array(array=w672, index (col)=0 ("disabled index (col)"), new element=w683) -> (w671:i32[][])  [unwired: 1 in]
                      n277 = Bundle By Name(cluster=w688, "Spliter_matrix"=w673, "Panel_matrix"=w671) -> (w685:T4)
                      n278 = Replace Array Subset(array=w687, new element=w685, index=w684) -> (w686:T4[])
                      n279 = global write "GVSNew View Global.vi" "DataView_Global"(w686) -> ()
                    }
                  }
                }
              }
            }
            frame "DOCK_M_LEFT" {
              n280 = stacked-sequence {
                seq-local: [_ w782 _ _ _ _] -> [_ _ w820 _ _ _]
                seq-local: [w713 _ _ _ _ _] -> [_ _ w819 _ _ _]
                seq-local: [_ w768 _ _ _ _] -> [_ _ _ _ w883 w906]
                seq-local: [_ w769 _ _ _ _] -> [_ _ _ _ w881 w907]
                seq-local: [_ w770 _ _ _ _] -> [_ _ _ _ w882 w908]
                seq-local: [_ w771 _ _ _ _] -> [_ _ _ _ w878 w909]
                seq-local: [_ w773 _ _ _ _] -> [_ _ w818 _ _ _]
                tunnel: w707 -> [_ _ w823 w854 _ _]
                tunnel: w706 -> [w718 w784 w822 w855 _ _]
                tunnel: w705 -> [w712 w774 _ _ _ _]
                tunnel: w704 -> [_ _ w825 _ _ _]
                tunnel: w703 -> [_ _ w824 _ _ _]
                tunnel: w702 -> [w719 _ _ _ _ _]
                tunnel: w701 -> [_ _ w817 w847 w877 w896]
                tunnel: w700 -> [_ _ _ w848 _ _]
                frame #0 {
                  n281 = Index Array(array=w712, index (row)=0, index (col)=0) -> (element=w709:i32)
                  n282 = Index Array(array=w718, index=w709) -> (element=w708:refnum<vi>)
                  n283 = property class="Bool"(reference=w708) -> ("Left"=w717:i32, "Top"=w716:i32)  [unwired: 1 in, 2 out]
                  n284 = call "GVSSearch Matrix Element.vi"("element"=w709, "index (row)"=0, "matrix in"=w719) -> ("index of element"=w720:i32)  [unwired: 8 in]
                  n285 = property class="Bool"(reference=w708) -> ("Height"=w714:u32, "Width"=w715:u32)  [unwired: 1 in, 2 out]
                  n286 = Greater Or Equal To 0?(x=w720) -> (x >= 0?=w721:bool)
                  n287 = case shown="True" w721 {
                    tunnel: w720 -> [_ w754]
                    tunnel: w719 -> [w724 w767]
                    tunnel: w712 -> [w732 w747]
                    tunnel: w717 -> [w742 w765]
                    tunnel: w716 -> [w741 w763]
                    tunnel: w715 -> [w740 w761]
                    tunnel: w714 -> [w739 w759]
                    tunnel: [w723 w753] -> w713
                    frame False {
                      (unwired) 1 ("index")
                      w737 = 0 ("index (col)")
                      n288 = Index Array(array=w732, index (row) #1=5 ("index (row)"), index (col) #1=w737, index (row) #2=6 ("index (row)"), index (col) #2=w737, index (row) #3=7 ("index (row)"), index (col) #3=w737, index (row) #4=8 ("index (row)"), index (col) #4=w737) -> (element #1=w731:i32, element #2=w730:i32, element #3=w729:i32, element #4=w728:i32)
                      n289 = Build Array(0 ("element"), w742, w741, w740, w739, w731, w730, w729, w728) -> (w725:u32[])
                      n290 = Array Size(array=w724) -> (size(s)=w726:i32[])
                      n291 = Index Array(array=w726) -> (element=w727:i32)  [unwired: 1 in]
                      n292 = Insert Into Array(array=w724, index (col)=w727, new element=w725) -> (w723:i32[][])  [unwired: 1 in]
                    }
                    frame True {
                      w752 = 0 ("index (col)")
                      n293 = Index Array(array=w747, index (row) #1=5 ("index (row)"), index (col) #1=w752, index (row) #2=6 ("index (row)"), index (col) #2=w752, index (row) #3=7 ("index (row)"), index (col) #3=w752, index (row) #4=8 ("index (row)"), index (col) #4=w752) -> (element #1=w746:i32, element #2=w745:i32, element #3=w744:i32, element #4=w743:i32)
                      n294 = Replace Array Subset(array=w767, new element #1=w765, index (row) #1=1 ("disabled index (row)"), index (col) #1=w754, new element #2=w763, index (row) #2=2 ("disabled index (row)"), index (col) #2=w754, new element #3=w761, index (row) #3=3 ("disabled index (row)"), index (col) #3=w754, new element #4=w759, index (row) #4=4 ("disabled index (row)"), index (col) #4=w754, new element #5=w746, index (row) #5=5 ("disabled index (row)"), index (col) #5=w754, new element #6=w745, index (row) #6=6 ("disabled index (row)"), index (col) #6=w754, new element #7=w744, index (row) #7=7 ("disabled index (row)"), index (col) #7=w754, new element #8=w743, index (row) #8=8 ("disabled index (row)"), index (col) #8=w754) -> (w753:i32[][])
                    }
                  }
                }
                frame #1 {
                  w779 = 0 ("index (col)")
                  n295 = Index Array(array=w774, index (row) #1=0 ("index (row)"), index (col) #1=w779, index (row) #2=1 ("index (row)"), index (col) #2=w779, index (row) #3=5 ("index (row)"), index (col) #3=w779, index (row) #4=6 ("index (row)"), index (col) #4=w779, index (row) #5=7 ("index (row)"), index (col) #5=w779, index (row) #6=8 ("index (row)"), index (col) #6=w779) -> (element #1=w773:i32, element #2=w772:i32, element #3=w771:i32, element #4=w770:i32, element #5=w769:i32, element #6=w768:i32)
                  n296 = Index Array(array=w784, index=w773) -> (element=w783:refnum<vi>)
                  n297 = case shown="2" w772 {
                    tunnel: w783 -> [_ w786 w816]
                    tunnel: w771 -> [_ w796 w808]
                    tunnel: w770 -> [_ _ _]
                    tunnel: w769 -> [_ w795 w809]
                    tunnel: w768 -> [_ _ _]
                    tunnel: w774 -> [w785 w794 w807]
                    tunnel: [w785 w791 w804] -> w782
                    frame 0, Default {
                    }
                    frame 2 {
                      w797 = 2 ("y")
                      n298 = Add(x=w796, y=w795) -> (x+y=w799:i32)
                      n299 = Subtract(x=w795, y=w796) -> (x-y=w798:i32)
                      n300 = Divide(x=w799, y=w797) -> (x/y=w790:dbl)
                      n301 = Divide(x=w798, y=w797) -> (x/y=w788:dbl)
                      n302 = To Long Integer(number=w790) -> (32bit integer=w789:i32)
                      n303 = To Long Integer(number=w788) -> (32bit integer=w787:i32)
                      n304 = Replace Array Subset(array=w794, new element=w789, index (row)=5 ("disabled index (row)"), index (col)=0) -> (w791:i32[][])
                      n305 = property class="Bool"(reference=w786, "Left"=w789) -> ()  [unwired: 1 in, 2 out]
                      n306 = property class="Bool"(reference=w786, "Width"=w787) -> ()  [unwired: 1 in, 2 out]
                    }
                    frame 1 {
                      n307 = Add(x=w809, y=w808) -> (x+y=w811:i32)
                      n308 = property class="Bool"(reference=w816) -> (reference out=w815:refnum<vi>, "Left"=w812:i32)  [unwired: 1 in, 1 out]
                      n309 = Divide(x=w811, y=2) -> (x/y=w801:dbl)
                      n310 = To Long Integer(number=w801) -> (32bit integer=w800:i32)
                      n311 = Replace Array Subset(array=w807, new element=w800, index (row)=5 ("disabled index (row)"), index (col)=0) -> (w804:i32[][])
                      n312 = Add(x=w812, y=w809) -> (x+y=w814:i32)
                      n313 = Divide(x=w814, y=2) -> (x/y=w803:dbl)
                      n314 = To Long Integer(number=w803) -> (32bit integer=w802:i32)
                      n315 = property class="Bool"(reference=w815, "Left"=w802) -> ()  [unwired: 1 in, 2 out]
                    }
                  }
                }
                frame #2 {
                  n316 = flat-sequence {
                    tunnel: w825 -> [w833]
                    tunnel: w824 -> [w831]
                    tunnel: w817 -> [w829]
                    tunnel: [w829] -> w821
                    tunnel: w820 -> [w828]
                    tunnel: w819 -> [w827]
                    tunnel: w818 -> [w826]
                    tunnel: w823 -> [w836]
                    tunnel: w822 -> [w835]
                    tunnel: w821 -> [w834]
                    frame #0 {
                      n317 = Bundle By Name(cluster=w833, "Selected_BarIdx"=w826, "Spliter_matrix"=w828, "split_pos_matrix"=w827) -> (w832:T4)
                      n318 = Replace Array Subset(array=w831, new element=w832, index=w829) -> (w830:T4[])
                      n319 = global write "GVSNew View Global.vi" "DataView_Global"(w830) -> ()
                    }
                    frame #1 {
                      n320 = flat-sequence {
                        tunnel: w836 -> [w841]
                        tunnel: w835 -> [w840]
                        tunnel: w834 -> [w842]
                        tunnel: [w842] -> w839
                        tunnel: [w841] -> w838
                        tunnel: [w840] -> w837
                        tunnel: w839 -> [w846]
                        tunnel: w838 -> [w845]
                        tunnel: w837 -> [w844]
                        frame #0 {
                          n321 = call "GVSResize Panel Current.vi"("DataView Array Idx"=w842, "close_panel"=TRUE, "spliter array"=w840, "SubPanel array"=w841) -> ()  [unwired: 8 in]
                        }
                        frame #1 {
                          n322 = call "GVSResize Panel Child.vi"("spliter array"=w844, "SubPanel array"=w845, "DataView Array Idx"=w846) -> ()  [unwired: 9 in]
                        }
                      }
                    }
                  }
                }
                frame #3 {
                  n323 = local read "cur_panel_idx"() -> (w850:i32)
                  n324 = call "GVSDataView Close Panel.vi"("Panel_Idx"=w850, "DataView Index"=w848) -> ("bResult"=w852:bool, "bHaveChild"=w853:bool, "closed_spliter_idx"=w849:i32)  [unwired: 7 in]
                  n325 = local write "spliter_idx"(w849) -> ()
                  n326 = And(x=w853, y=w852) -> (x .and. y?=w851:bool)
                  n327 = case shown="True" w851 {
                    tunnel: w854 -> [_ w861]
                    tunnel: w855 -> [_ w860]
                    tunnel: w847 -> [_ w859]
                    frame False {
                    }
                    frame True {
                      n328 = flat-sequence {
                        tunnel: w861 -> [w863]
                        tunnel: w860 -> [w862]
                        tunnel: w859 -> [w864]
                        tunnel: [w864] -> w858
                        tunnel: [w863] -> w857
                        tunnel: [w862] -> w856
                        tunnel: w858 -> [w868]
                        tunnel: w857 -> [w867]
                        tunnel: w856 -> [w866]
                        frame #0 {
                          n329 = call "GVSResize Panel Current.vi"("DataView Array Idx"=w864, "close_panel"=TRUE, "spliter array"=w862, "SubPanel array"=w863) -> ()  [unwired: 8 in]
                        }
                        frame #1 {
                          n330 = call "GVSResize Panel Child.vi"("spliter array"=w866, "SubPanel array"=w867, "DataView Array Idx"=w868) -> ()  [unwired: 9 in]
                        }
                      }
                    }
                  }
                }
                frame #4 {
                  n331 = global read "GVSNew View Global.vi" "DataView_Global"() -> (w893:T4[])
                  n332 = Index Array(array=w893, index=w877) -> (element=w892:T4)
                  n333 = Unbundle By Name(w892) -> ("Spliter Ref Array"=w891:refnum<vi>[], "Panel Ref Array"=w890:refnum<vi>[])  [unwired: 1 out]
                  n334 = Add(x=w881, y=w878) -> (x+y=w886:i32)
                  n335 = global read "GVSNew View Global.vi" "splitter_thickness"() -> (w869:u32)
                  n336 = Divide(x=w886, y=2) -> (x/y=w876:dbl)
                  n337 = To Long Integer(number=w876) -> (32bit integer=w875:i32)
                  n338 = local read "cur_panel_idx"() -> (w889:i32)
                  n339 = Subtract(x=w875, y=w869) -> (x-y=w879:u32)
                  n340 = Subtract(x=w879, y=w878) -> (x-y=w884:u32)
                  n341 = global read "GVSNew View Global.vi" "panel_offset"() -> (w871:i32)
                  n342 = local read "spliter_idx"() -> (w895:i32)
                  n343 = Subtract(x=w883, y=w882) -> (x-y=w880:i32)
                  n344 = Index Array(array=w891, index=w895) -> (element=w874:refnum<vi>)
                  n345 = Index Array(array=w890, index=w889) -> (element=w888:refnum<vi>)
                  n346 = Subtract(x=w878, y=w871) -> (x-y=w873:i32)
                  n347 = Subtract(x=w882, y=w871) -> (x-y=w872:i32)
                  n348 = property class="SubPnl"(reference=w888, "Left"=w873, "Top"=w872, "Height"=w880, "Width"=w884, "Visible"=TRUE) -> ()  [unwired: 1 in, 2 out]
                  n349 = property class="Bool"(reference=w874, "Left"=w879, "Top"=w882, "Visible"=TRUE) -> ()  [unwired: 1 in, 2 out]
                  n350 = global read "GVSNew View Global.vi" "splitter_thickness"() -> (w870:u32)
                  n351 = property class="Bool"(reference=w874, "Height"=w880, "Width"=w870) -> ()  [unwired: 1 in, 2 out]
                }
                frame #5 {
                  n352 = global read "GVSNew View Global.vi" "DataView_Global"() -> (w898:T4[])
                  n353 = Index Array(array=w898, index=w896) -> (element=w899:T4)
                  n354 = Unbundle By Name(w899) -> ("Spliter_matrix"=w905:i32[][], "Panel_matrix"=w900:i32[][], "child_spliterIdx_matrix"=w897:i32[][])  [unwired: 1 out]
                  n355 = Index Array(array=w905, index (row)=0) -> (element=w903:i32[])  [unwired: 1 in]
                  n356 = Array Size(array=w903) -> (size(s)=w902:i32)
                  n357 = Greater Than 0?(x=w902) -> (x > 0?=w901:bool)
                  n358 = case shown="True" w901 {
                    tunnel: w897 -> [w951 _]
                    tunnel: w909 -> [w945 w977]
                    tunnel: w908 -> [w944 w976]
                    tunnel: w907 -> [w943 w975]
                    tunnel: w906 -> [w942 w974]
                    tunnel: w905 -> [w918 w955]
                    tunnel: w900 -> [w911 w961]
                    tunnel: w897 -> [w926 _]
                    tunnel: w899 -> [w934 w969]
                    tunnel: w898 -> [w933 w968]
                    tunnel: w896 -> [w930 w965]
                    frame True {
                      w946 = -1 ("element")
                      w915 = 0 ("index (col)")
                      w922 = 0 ("index (col)")
                      n359 = Index Array(array=w918, index (row) #1=0 ("index (row)"), index (col) #1=w922, index (row) #2=3 ("index (row)"), index (col) #2=w922) -> (element #1=w920:i32, element #2=w921:i32)
                      n360 = local write "child_sp_count"(w921) -> ()
                      n361 = Index Array(array=w951, index (col)=w920) -> (element=w937:i32[])  [unwired: 1 in]
                      n362 = local read "child_sp_count"() -> (w948:i32)
                      n363 = Insert Into Array(array=w937, index=0, new element=w920) -> (w935:i32[])
                      n364 = Increment(x=w948) -> (x+1=w947:i32)
                      n365 = local read "spliter_idx"() -> (w917:i32)
                      n366 = local read "spliter_idx"() -> (w940:i32)
                      n367 = local read "cur_panel_idx"() -> (w939:i32)
                      n368 = Build Array(w940, 1 ("element"), w946, w947, w946, w945, w944, w943, w942) -> (w941:i32[])
                      n369 = Replace Array Subset(array=w918, new element #1=w917, index (row) #1=2 ("disabled index (row)"), index (col) #1=w915, new element #2=2 ("new element/submatrix"), index (row) #2=4 ("disabled index (row)"), index (col) #2=w915) -> (w913:i32[][])
                      n370 = Insert Into Array(array=w913, index (col)=0 ("disabled index (col)"), new element=w941) -> (w912:i32[][])  [unwired: 1 in]
                      n371 = Build Array(w940, w939, 1 ("element")) -> (w929:i32[])
                      n372 = local read "spliter_idx"() -> (w927:i32)
                      n373 = Insert Into Array(array=w911, index (col)=0 ("disabled index (col)"), new element=w929) -> (w910:i32[][])  [unwired: 1 in]
                      n374 = Replace Array Subset(array=w926, new element=w935, index (col)=w927) -> (w925:i32[][])  [unwired: 1 in]
                      n375 = Bundle By Name(cluster=w934, "Spliter_matrix"=w912, "Panel_matrix"=w910, "child_spliterIdx_matrix"=w925) -> (w931:T4)
                      n376 = Replace Array Subset(array=w933, new element=w931, index=w930) -> (w932:T4[])
                      n377 = global write "GVSNew View Global.vi" "DataView_Global"(w932) -> ()
                    }
                    frame False {
                      w956 = 0 ("index (col)")
                      w978 = -1 ("element")
                      n378 = local read "spliter_idx"() -> (w957:i32)
                      n379 = Replace Array Subset(array=w961, new element #1=w957, index (row) #1=0 ("disabled index (row)"), index (col) #1=w956, new element #2=2 ("new element/submatrix"), index (row) #2=2 ("disabled index (row)"), index (col) #2=w956) -> (w953:i32[][])
                      n380 = local read "spliter_idx"() -> (w972:i32)
                      n381 = local read "cur_panel_idx"() -> (w971:i32)
                      n382 = Build Array(w972, 1 ("element"), w978, 0 ("element"), w978, w977, w976, w975, w974) -> (w973:i32[])
                      n383 = Insert Into Array(array=w955, index (col)=0 ("disabled index (col)"), new element=w973) -> (w954:i32[][])  [unwired: 1 in]
                      n384 = Build Array(w972, w971, 1 ("element")) -> (w964:i32[])
                      n385 = Insert Into Array(array=w953, index (col)=0 ("disabled index (col)"), new element=w964) -> (w952:i32[][])  [unwired: 1 in]
                      n386 = Bundle By Name(cluster=w969, "Spliter_matrix"=w954, "Panel_matrix"=w952) -> (w966:T4)
                      n387 = Replace Array Subset(array=w968, new element=w966, index=w965) -> (w967:T4[])
                      n388 = global write "GVSNew View Global.vi" "DataView_Global"(w967) -> ()
                    }
                  }
                }
              }
            }
            frame "DOCK_M_RIGHT" {
              n389 = stacked-sequence {
                seq-local: [_ w1063 _ _ _ _] -> [_ _ w1100 _ _ _]
                seq-local: [w994 _ _ _ _ _] -> [_ _ w1099 _ _ _]
                seq-local: [_ w1049 _ _ _ _] -> [_ _ _ _ w1163 w1186]
                seq-local: [_ w1050 _ _ _ _] -> [_ _ _ _ w1158 w1187]
                seq-local: [_ w1051 _ _ _ _] -> [_ _ _ _ w1162 w1188]
                seq-local: [_ w1052 _ _ _ _] -> [_ _ _ _ w1160 w1189]
                seq-local: [_ w1054 _ _ _ _] -> [_ _ w1098 _ _ _]
                tunnel: w982 -> [_ _ _ w1127 _ _]
                tunnel: w988 -> [_ _ w1103 w1134 _ _]
                tunnel: w987 -> [w999 w1065 w1102 w1135 _ _]
                tunnel: w986 -> [w992 w1055 _ _ _ _]
                tunnel: w985 -> [_ _ w1105 _ _ _]
                tunnel: w984 -> [_ _ w1104 _ _ _]
                tunnel: w983 -> [w1000 _ _ _ _ _]
                tunnel: w981 -> [_ _ w1097 w1128 w1157 w1176]
                frame #0 {
                  n390 = Index Array(array=w992, index (row)=0, index (col)=0) -> (element=w990:i32)
                  n391 = Index Array(array=w999, index=w990) -> (element=w989:refnum<vi>)
                  n392 = property class="Bool"(reference=w989) -> ("Left"=w998:i32, "Top"=w997:i32)  [unwired: 1 in, 2 out]
                  n393 = call "GVSSearch Matrix Element.vi"("element"=w990, "index (row)"=0, "matrix in"=w1000) -> ("index of element"=w1001:i32)  [unwired: 8 in]
                  n394 = property class="Bool"(reference=w989) -> ("Height"=w995:u32, "Width"=w996:u32)  [unwired: 1 in, 2 out]
                  n395 = Greater Or Equal To 0?(x=w1001) -> (x >= 0?=w1002:bool)
                  n396 = case shown="True" w1002 {
                    tunnel: w1001 -> [_ w1035]
                    tunnel: w1000 -> [w1005 w1048]
                    tunnel: w992 -> [w1013 w1029]
                    tunnel: w998 -> [w1023 w1046]
                    tunnel: w997 -> [w1022 w1044]
                    tunnel: w996 -> [w1021 w1042]
                    tunnel: w995 -> [w1020 w1040]
                    tunnel: [w1004 w1024] -> w994
                    frame False {
                      (unwired) 1 ("index")
                      w1018 = 0 ("index (col)")
                      n397 = Index Array(array=w1013, index (row) #1=5 ("index (row)"), index (col) #1=w1018, index (row) #2=6 ("index (row)"), index (col) #2=w1018, index (row) #3=7 ("index (row)"), index (col) #3=w1018, index (row) #4=8 ("index (row)"), index (col) #4=w1018) -> (element #1=w1012:i32, element #2=w1011:i32, element #3=w1010:i32, element #4=w1009:i32)
                      n398 = Build Array(0 ("element"), w1023, w1022, w1021, w1020, w1012, w1011, w1010, w1009) -> (w1006:u32[])
                      n399 = Array Size(array=w1005) -> (size(s)=w1007:i32[])
                      n400 = Index Array(array=w1007) -> (element=w1008:i32)  [unwired: 1 in]
                      n401 = Insert Into Array(array=w1005, index (col)=w1008, new element=w1006) -> (w1004:i32[][])  [unwired: 1 in]
                    }
                    frame True {
                      w1034 = 0 ("index (col)")
                      n402 = Index Array(array=w1029, index (row) #1=5 ("index (row)"), index (col) #1=w1034, index (row) #2=6 ("index (row)"), index (col) #2=w1034, index (row) #3=7 ("index (row)"), index (col) #3=w1034, index (row) #4=8 ("index (row)"), index (col) #4=w1034) -> (element #1=w1028:i32, element #2=w1027:i32, element #3=w1026:i32, element #4=w1025:i32)
                      n403 = Replace Array Subset(array=w1048, new element #1=w1046, index (row) #1=1 ("disabled index (row)"), index (col) #1=w1035, new element #2=w1044, index (row) #2=2 ("disabled index (row)"), index (col) #2=w1035, new element #3=w1042, index (row) #3=3 ("disabled index (row)"), index (col) #3=w1035, new element #4=w1040, index (row) #4=4 ("disabled index (row)"), index (col) #4=w1035, new element #5=w1028, index (row) #5=5 ("disabled index (row)"), index (col) #5=w1035, new element #6=w1027, index (row) #6=6 ("disabled index (row)"), index (col) #6=w1035, new element #7=w1026, index (row) #7=7 ("disabled index (row)"), index (col) #7=w1035, new element #8=w1025, index (row) #8=8 ("disabled index (row)"), index (col) #8=w1035) -> (w1024:i32[][])
                    }
                  }
                }
                frame #1 {
                  w1060 = 0 ("index (col)")
                  n404 = Index Array(array=w1055, index (row) #1=0 ("index (row)"), index (col) #1=w1060, index (row) #2=1 ("index (row)"), index (col) #2=w1060, index (row) #3=5 ("index (row)"), index (col) #3=w1060, index (row) #4=6 ("index (row)"), index (col) #4=w1060, index (row) #5=7 ("index (row)"), index (col) #5=w1060, index (row) #6=8 ("index (row)"), index (col) #6=w1060) -> (element #1=w1054:i32, element #2=w1053:i32, element #3=w1052:i32, element #4=w1051:i32, element #5=w1050:i32, element #6=w1049:i32)
                  n405 = Index Array(array=w1065, index=w1054) -> (element=w1064:refnum<vi>)
                  n406 = case shown="2" w1053 {
                    tunnel: w1064 -> [_ w1067 w1096]
                    tunnel: w1052 -> [_ w1075 w1088]
                    tunnel: w1051 -> [_ _ _]
                    tunnel: w1050 -> [_ w1076 w1089]
                    tunnel: w1049 -> [_ _ _]
                    tunnel: w1055 -> [w1066 w1074 w1084]
                    tunnel: [w1066 w1070 w1080] -> w1063
                    frame 0, Default {
                    }
                    frame 2 {
                      w1077 = 2 ("y")
                      n407 = Add(x=w1075, y=w1076) -> (x+y=w1079:i32)
                      n408 = Subtract(x=w1076, y=w1075) -> (x-y=w1078:i32)
                      n409 = Divide(x=w1079, y=w1077) -> ()  [unwired: 1 out]
                      n410 = Divide(x=w1078, y=w1077) -> (x/y=w1069:dbl)
                      n411 = To Long Integer(number=w1069) -> (32bit integer=w1068:i32)
                      n412 = Add(x=w1075, y=w1068) -> (x+y=w1071:i32)
                      n413 = Replace Array Subset(array=w1074, new element=w1071, index (row)=7 ("disabled index (row)"), index (col)=0) -> (w1070:i32[][])
                      n414 = property class="Bool" props=["Left"](reference=w1067) -> ()  [unwired: 1 in, 3 out]
                      n415 = property class="Bool"(reference=w1067, "Width"=w1068) -> ()  [unwired: 1 in, 2 out]
                    }
                    frame 1 {
                      n416 = Add(x=w1089, y=w1088) -> (x+y=w1091:i32)
                      n417 = property class="Bool"(reference=w1096) -> (reference out=w1095:refnum<vi>, "Left"=w1092:i32)  [unwired: 1 in, 1 out]
                      n418 = Divide(x=w1091, y=2) -> (x/y=w1085:dbl)
                      n419 = To Long Integer(number=w1085) -> (32bit integer=w1081:i32)
                      n420 = Replace Array Subset(array=w1084, new element=w1081, index (row)=7 ("disabled index (row)"), index (col)=0) -> (w1080:i32[][])
                      n421 = Add(x=w1092, y=w1088) -> (x+y=w1094:i32)
                      n422 = Divide(x=w1094, y=2) -> (x/y=w1087:dbl)
                      n423 = To Long Integer(number=w1087) -> (32bit integer=w1086:i32)
                      n424 = property class="Bool"(reference=w1095, "Left"=w1086) -> ()  [unwired: 1 in, 2 out]
                    }
                  }
                }
                frame #2 {
                  n425 = flat-sequence {
                    tunnel: w1105 -> [w1113]
                    tunnel: w1104 -> [w1111]
                    tunnel: w1097 -> [w1109]
                    tunnel: [w1109] -> w1101
                    tunnel: w1100 -> [w1108]
                    tunnel: w1099 -> [w1107]
                    tunnel: w1098 -> [w1106]
                    tunnel: w1103 -> [w1116]
                    tunnel: w1102 -> [w1115]
                    tunnel: w1101 -> [w1114]
                    frame #0 {
                      n426 = Bundle By Name(cluster=w1113, "Selected_BarIdx"=w1106, "Spliter_matrix"=w1108, "split_pos_matrix"=w1107) -> (w1112:T4)
                      n427 = Replace Array Subset(array=w1111, new element=w1112, index=w1109) -> (w1110:T4[])
                      n428 = global write "GVSNew View Global.vi" "DataView_Global"(w1110) -> ()
                    }
                    frame #1 {
                      n429 = flat-sequence {
                        tunnel: w1116 -> [w1121]
                        tunnel: w1115 -> [w1120]
                        tunnel: w1114 -> [w1122]
                        tunnel: [w1122] -> w1119
                        tunnel: [w1121] -> w1118
                        tunnel: [w1120] -> w1117
                        tunnel: w1119 -> [w1126]
                        tunnel: w1118 -> [w1125]
                        tunnel: w1117 -> [w1124]
                        frame #0 {
                          n430 = call "GVSResize Panel Current.vi"("DataView Array Idx"=w1122, "close_panel"=TRUE, "spliter array"=w1120, "SubPanel array"=w1121) -> ()  [unwired: 8 in]
                        }
                        frame #1 {
                          n431 = call "GVSResize Panel Child.vi"("spliter array"=w1124, "SubPanel array"=w1125, "DataView Array Idx"=w1126) -> ()  [unwired: 9 in]
                        }
                      }
                    }
                  }
                }
                frame #3 {
                  n432 = local read "cur_panel_idx"() -> (w1130:i32)
                  n433 = call "GVSDataView Close Panel.vi"("Panel_Idx"=w1130, "DataView Index"=w1127) -> ("bResult"=w1132:bool, "bHaveChild"=w1133:bool, "closed_spliter_idx"=w1129:i32)  [unwired: 7 in]
                  n434 = And(x=w1133, y=w1132) -> (x .and. y?=w1131:bool)
                  n435 = local write "spliter_idx"(w1129) -> ()
                  n436 = case shown="True" w1131 {
                    tunnel: w1134 -> [_ w1141]
                    tunnel: w1135 -> [_ w1140]
                    tunnel: w1128 -> [_ w1139]
                    frame False {
                    }
                    frame True {
                      n437 = flat-sequence {
                        tunnel: w1141 -> [w1143]
                        tunnel: w1140 -> [w1142]
                        tunnel: w1139 -> [w1144]
                        tunnel: [w1144] -> w1138
                        tunnel: [w1143] -> w1137
                        tunnel: [w1142] -> w1136
                        tunnel: w1138 -> [w1148]
                        tunnel: w1137 -> [w1147]
                        tunnel: w1136 -> [w1146]
                        frame #0 {
                          n438 = call "GVSResize Panel Current.vi"("DataView Array Idx"=w1144, "close_panel"=TRUE, "spliter array"=w1142, "SubPanel array"=w1143) -> ()  [unwired: 8 in]
                        }
                        frame #1 {
                          n439 = call "GVSResize Panel Child.vi"("spliter array"=w1146, "SubPanel array"=w1147, "DataView Array Idx"=w1148) -> ()  [unwired: 9 in]
                        }
                      }
                    }
                  }
                }
                frame #4 {
                  n440 = global read "GVSNew View Global.vi" "DataView_Global"() -> (w1173:T4[])
                  n441 = Index Array(array=w1173, index=w1157) -> (element=w1172:T4)
                  n442 = Unbundle By Name(w1172) -> ("Spliter Ref Array"=w1171:refnum<vi>[], "Panel Ref Array"=w1170:refnum<vi>[])  [unwired: 1 out]
                  n443 = Add(x=w1158, y=w1160) -> (x+y=w1166:i32)
                  n444 = global read "GVSNew View Global.vi" "splitter_thickness"() -> (w1149:u32)
                  n445 = Divide(x=w1166, y=2) -> (x/y=w1156:dbl)
                  n446 = To Long Integer(number=w1156) -> (32bit integer=w1155:i32)
                  n447 = local read "cur_panel_idx"() -> (w1169:i32)
                  n448 = global read "GVSNew View Global.vi" "panel_offset"() -> (w1151:i32)
                  n449 = Add(x=w1155, y=w1149) -> (x+y=w1159:u32)
                  n450 = Subtract(x=w1158, y=w1159) -> (x-y=w1164:u32)
                  n451 = local read "spliter_idx"() -> (w1175:i32)
                  n452 = Subtract(x=w1163, y=w1162) -> (x-y=w1161:i32)
                  n453 = Index Array(array=w1171, index=w1175) -> (element=w1154:refnum<vi>)
                  n454 = Index Array(array=w1170, index=w1169) -> (element=w1168:refnum<vi>)
                  n455 = Subtract(x=w1159, y=w1151) -> (x-y=w1153:u32)
                  n456 = Subtract(x=w1162, y=w1151) -> (x-y=w1152:i32)
                  n457 = property class="SubPnl"(reference=w1168, "Left"=w1153, "Top"=w1152, "Height"=w1161, "Width"=w1164, "Visible"=TRUE) -> ()  [unwired: 1 in, 2 out]
                  n458 = property class="Bool"(reference=w1154, "Left"=w1155, "Top"=w1162, "Visible"=TRUE) -> ()  [unwired: 1 in, 2 out]
                  n459 = global read "GVSNew View Global.vi" "splitter_thickness"() -> (w1150:u32)
                  n460 = property class="Bool"(reference=w1154, "Height"=w1161, "Width"=w1150) -> ()  [unwired: 1 in, 2 out]
                }
                frame #5 {
                  n461 = global read "GVSNew View Global.vi" "DataView_Global"() -> (w1178:T4[])
                  n462 = Index Array(array=w1178, index=w1176) -> (element=w1179:T4)
                  n463 = Unbundle By Name(w1179) -> ("Spliter_matrix"=w1185:i32[][], "Panel_matrix"=w1180:i32[][], "child_spliterIdx_matrix"=w1177:i32[][])  [unwired: 1 out]
                  n464 = Index Array(array=w1185, index (row)=0) -> (element=w1183:i32[])  [unwired: 1 in]
                  n465 = Array Size(array=w1183) -> (size(s)=w1182:i32)
                  n466 = Greater Than 0?(x=w1182) -> (x > 0?=w1181:bool)
                  n467 = case shown="True" w1181 {
                    tunnel: w1177 -> [w1231 _]
                    tunnel: w1189 -> [w1225 w1257]
                    tunnel: w1188 -> [w1224 w1256]
                    tunnel: w1187 -> [w1223 w1255]
                    tunnel: w1186 -> [w1222 w1254]
                    tunnel: w1185 -> [w1200 w1235]
                    tunnel: w1180 -> [w1192 w1241]
                    tunnel: w1177 -> [w1207 _]
                    tunnel: w1179 -> [w1214 w1249]
                    tunnel: w1178 -> [w1213 w1248]
                    tunnel: w1176 -> [w1190 w1245]
                    frame True {
                      w1226 = -1 ("element")
                      w1197 = 0 ("index (col)")
                      w1203 = 0 ("index (col)")
                      n468 = Index Array(array=w1200, index (row) #1=0 ("index (row)"), index (col) #1=w1203, index (row) #2=3 ("index (row)"), index (col) #2=w1203) -> (element #1=w1201:i32, element #2=w1202:i32)
                      n469 = local write "child_sp_count"(w1202) -> ()
                      n470 = Index Array(array=w1231, index (col)=w1201) -> (element=w1217:i32[])  [unwired: 1 in]
                      n471 = local read "child_sp_count"() -> (w1228:i32)
                      n472 = Insert Into Array(array=w1217, index=0, new element=w1201) -> (w1215:i32[])
                      n473 = Increment(x=w1228) -> (x+1=w1227:i32)
                      n474 = local read "spliter_idx"() -> (w1198:i32)
                      n475 = local read "spliter_idx"() -> (w1220:i32)
                      n476 = local read "cur_panel_idx"() -> (w1219:i32)
                      n477 = Build Array(w1220, 1 ("element"), w1226, w1227, w1226, w1225, w1224, w1223, w1222) -> (w1221:i32[])
                      n478 = Replace Array Subset(array=w1200, new element #1=w1198, index (row) #1=2 ("disabled index (row)"), index (col) #1=w1197, new element #2=1 ("new element/submatrix"), index (row) #2=4 ("disabled index (row)"), index (col) #2=w1197) -> (w1194:i32[][])
                      n479 = Insert Into Array(array=w1194, index (col)=0 ("disabled index (col)"), new element=w1221) -> (w1193:i32[][])  [unwired: 1 in]
                      n480 = Build Array(w1220, w1219, 2 ("element")) -> (w1210:i32[])
                      n481 = local read "spliter_idx"() -> (w1208:i32)
                      n482 = Insert Into Array(array=w1192, index (col)=0 ("disabled index (col)"), new element=w1210) -> (w1191:i32[][])  [unwired: 1 in]
                      n483 = Replace Array Subset(array=w1207, new element=w1215, index (col)=w1208) -> (w1206:i32[][])  [unwired: 1 in]
                      n484 = Bundle By Name(cluster=w1214, "Spliter_matrix"=w1193, "Panel_matrix"=w1191, "child_spliterIdx_matrix"=w1206) -> (w1211:T4)
                      n485 = Replace Array Subset(array=w1213, new element=w1211, index=w1190) -> (w1212:T4[])
                      n486 = global write "GVSNew View Global.vi" "DataView_Global"(w1212) -> ()
                    }
                    frame False {
                      w1236 = 0 ("index (col)")
                      w1258 = -1 ("element")
                      n487 = local read "spliter_idx"() -> (w1239:i32)
                      n488 = Replace Array Subset(array=w1241, new element #1=w1239, index (row) #1=0 ("disabled index (row)"), index (col) #1=w1236, new element #2=1 ("new element/submatrix"), index (row) #2=2 ("disabled index (row)"), index (col) #2=w1236) -> (w1233:i32[][])
                      n489 = local read "spliter_idx"() -> (w1252:i32)
                      n490 = local read "cur_panel_idx"() -> (w1251:i32)
                      n491 = Build Array(w1252, 1 ("element"), w1258, 0 ("element"), w1258, w1257, w1256, w1255, w1254) -> (w1253:i32[])
                      n492 = Insert Into Array(array=w1235, index (col)=0 ("disabled index (col)"), new element=w1253) -> (w1234:i32[][])  [unwired: 1 in]
                      n493 = Build Array(w1252, w1251, 2 ("element")) -> (w1244:i32[])
                      n494 = Insert Into Array(array=w1233, index (col)=0 ("disabled index (col)"), new element=w1244) -> (w1232:i32[][])  [unwired: 1 in]
                      n495 = Bundle By Name(cluster=w1249, "Spliter_matrix"=w1234, "Panel_matrix"=w1232) -> (w1246:T4)
                      n496 = Replace Array Subset(array=w1248, new element=w1246, index=w1245) -> (w1247:T4[])
                      n497 = global write "GVSNew View Global.vi" "DataView_Global"(w1247) -> ()
                    }
                  }
                }
              }
            }
          }
          n498 = local write "cur_panel_idx"(w139) -> ()
        }
      }
    }
    frame #1 {
      n499 = global read "GVSNew View Global.vi" "DataView_Global"() -> (w1266:T4[])
      n500 = call "GVSGet DataView Arrary Idx.vi"("DataView Idx In"=w1261) -> ("DataView Arrary Idx out"=w1262:i32)  [unwired: 10 in]
      n501 = flat-sequence {
        tunnel: w1263 -> [w1272]
        tunnel: w1264 -> [w1269]
        tunnel: w1261 -> [w1270]
        frame #0 {
          w1268 = 0 ("index (row)")
          n502 = Index Array(array=w1269, index (row)=w1268, index (col)=w1268) -> (element=w1267:i32)
          n503 = Index Array(array=w1272, index=w1267) -> (element=w1271:refnum<vi>)
          n504 = call "GVSDataView Splitter MDown Process.vi"("DataView Index"=w1270, "Selected Spliter Ref"=w1271) -> ()  [unwired: 9 in, 1 out]
        }
      }
      n505 = Index Array(array=w1266, index=w1262) -> (element=w1265:T4)
      n506 = Unbundle By Name(w1265) -> ("Spliter_matrix"=w1264:i32[][], "Spliter Ref Array"=w1263:refnum<vi>[])
    }
  }
